vi "test_Parse FPGA Bitfile.vi"(8 "error in (no error)":errorcluster) -> (0 "error out":errorcluster)   [LabVIEW 2018, in "Load And Parse Bitfile Testing.lvclass"]
uses:
  Load And Parse Bitfile Testing.lvclass
  <vilib>/rvi/Bitfile/nirviControlStructure.ctl
  <vilib>/rvi/Bitfile/nirviTypdefDescription.ctl
  <vilib>/rvi/Bitfile/nirviMechanicalAction.ctl
  <vilib>/rvi/Bitfile/nirviSubControlStructure.ctl
  <vilib>/rvi/Bitfile/nirviClusterElementControl.ctl
  <vilib>/rvi/FIFO/Fifo_Types/Fifo_DMA_Config.ctl
  <vilib>/rvi/DataTransferAndStorage/Container/Common/niFpgaDataTypeControl.ctl
  <vilib>/rvi/ClientSDK/Core/ModuleGeneration/CommunicationInterfaceUtility/niFpgaDmaChannelImplementation.ctl
  <vilib>/addons/_JKI Toolkits/VI Tester/TestCase.llb/TestCase.lvclass
  Addon/Addon System Explorer/FPGA Addon System Explorer.lvlib
  C:/Program Files (x86)/National Instruments/LabVIEW 2018/vi.lib/addons/_JKI Toolkits/VI Tester/TestCase.llb/TestCase.lvclass
panel:
  out "TestCase out":refnum<class "Load And Parse Bitfile Testing.lvclass">
  in  "TestCase in":refnum<class "Load And Parse Bitfile Testing.lvclass">
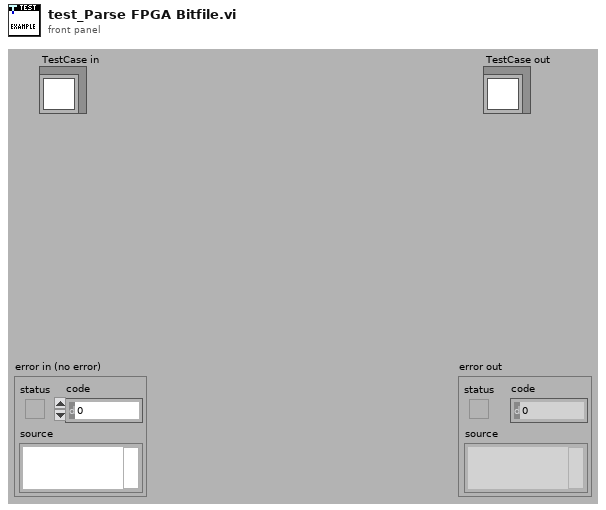
[diagram p1: front panel]
types:
  T1 = typedef "Fifo_DMA_Config.ctl" = cluster{"Name":string, "Depth":u32, "Write? (Deprecated:Use Implementation)":bool, "Physical Channel":u32, "Base Address":u32, "Data Width":u32, "Data Type":T2, "FXP Properties":variant, "Write Window Address":u32, "Implementation":T3, "Control Set":u32}
  T2 = typedef "niFpgaDataTypeControl.ctl" = enum32{"Boolean", "I8", "I16", "I32", "I64", "U8", "U16", "U32", "U64", "FXP", "CustomControl", "SGL"}
  T3 = typedef "niFpgaDmaChannelImplementation.ctl" = enum16{"niFpgaTargetToHost", "niFpgaHostToTarget", "niFpgaPeerToPeerWriter", "niFpgaPeerToPeerReader", "niCoreTargetToHost", "niCoreHostToTarget"}
  T4 = typedef "nirviControlStructure.ctl" = cluster{"Name":string, "Hidden":bool, "Indicator":bool, "Flattened Type":string, "Grouping":cluster{"Grouped":bool, "Member Names":string[], "Member IDs":u32[]}, "Address":u32, "Size":u32, "Class":u32, "Internal":bool, "Typedef":T5, "ID":u32, "Bidirectional":bool, "Synchronous":bool, "Mechanical Action":T6, "Sub Controls":T7[], "Access May Timeout":bool, "Register Node":bool}
  T5 = typedef "nirviTypdefDescription.ctl" = cluster{"Typedef":bool, "Path":path}
  T6 = typedef "nirviMechanicalAction.ctl" = enum8{"Switch When Pressed", "Switch When Released", "Switch Until Released", "Latch When Pressed", "Latch When Released", "Latch Until Released"}
  T7 = typedef "nirviSubControlStructure.ctl" = cluster{"Name":string, "flattened Type":string, "Cluster Information":T8, "Typedef":T5}
  T8 = typedef "nirviClusterElementControl.ctl" = cluster{"Name Hierarchy":string[], "Item Order":u32[]}
  T9 = typedef "niFpgaBitfileStructure_VI.ctl" = cluster{"Name":string, "RegisterMap":T4[], "Icon":T10}
  T10 = typedef "imagedata.ctl" = cluster{"image type":i32, "image depth":i32, "image":u8[], "mask":u8[], "colors":u32[], "Rectangle":cluster{"left":i16, "top":i16, "right":i16, "bottom":i16}}
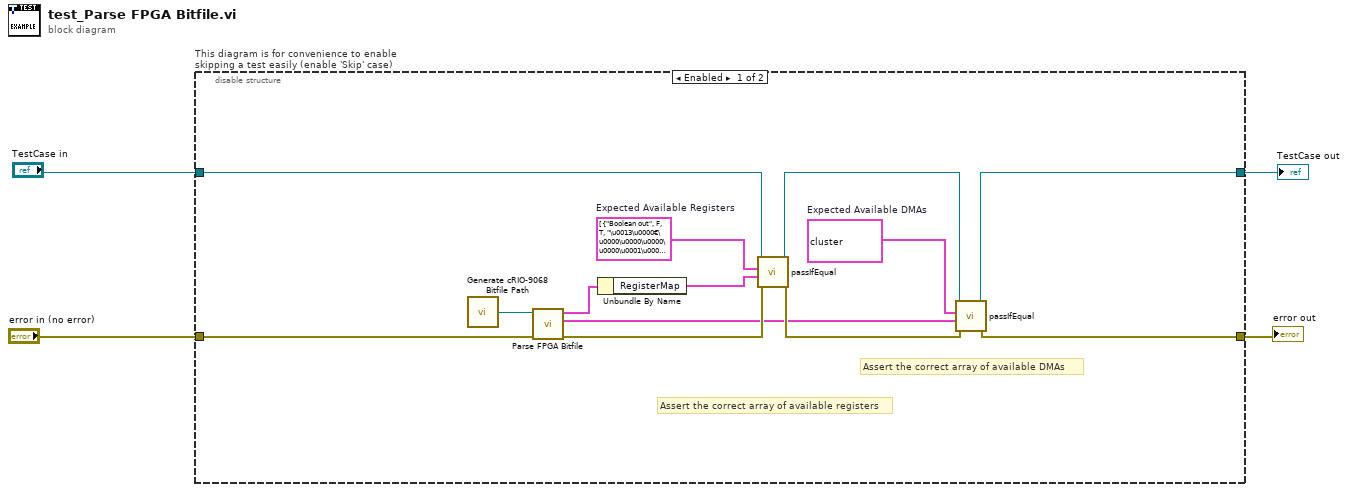
[diagram p0: block diagram]
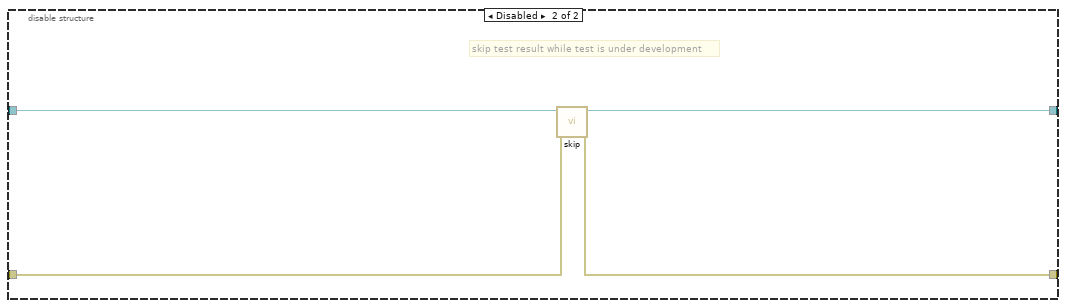
[diagram p2: hidden frame]
diagram:
  n1 = disable-structure "This diagram is for convenience to enable skipping a test easily (enable 'Skip' case)" shown="Enabled" {
    disable-tunnel: "TestCase in" -> [w17 w21]
    disable-tunnel: [w12 w19] -> w1
    disable-tunnel: [w10 w20] -> w3
    disable-tunnel: "error in (no error)" -> [w16 w18]
    frame Enabled {
      w7 = T1[] [{"Name"="Slow", "Depth"=1023, "Write? (Deprecated:Use Implementation)"=TRUE, "Physical Channel"=0, "Base Address"=65472, "Data Width"=32, "Data Type"=enum."SGL", "FXP Properties"=variant(fxp<+/-,32,0> 0.0), "Write Window Address"=0, "Implementation"=enum."niFpgaTargetToHost", "Control Set"=0}, {"Name"="Medium", "Depth"=1023, "Write? (Deprecated:Use Implementation)"=TRUE, "Physical Channel"=1, "Base Address"=65408, "Data Width"=32, "Data Type"=enum."SGL", "FXP Properties"=variant(fxp<+/-,32,0> 0.0), "Write Window Address"=0, "Implementation"=enum."niFpgaTargetToHost", "Control Set"=1}, {"Name"="HostToTarget2", "Depth"=1029, "Write? (Deprecated:Use Implementation)"=FALSE, "Physical Channel"=2, "Base Address"=65344, "Data Width"=32, "Data Type"=enum."SGL", "FXP Properties"=variant(fxp<+/-,32,0> 0.0), "Write Window Address"=0, "Implementation"=enum."niFpgaHostToTarget", "Control Set"=2}, {"Name"="HostToTarget1", "Depth"=1029, "Write? (Deprecated:Use Implementation)"=FALSE, "Physical Channel"=3, "Base Address"=65280, "Data Width"=32, "Data Type"=enum."SGL", "FXP Properties"=variant(fxp<+/-,32,0> 0.0), "Write Window Address"=0, "Implementation"=enum."niFpgaHostToTarget", "Control Set"=3}, {"Name"="Fast", "Depth"=1023, "Write? (Deprecated:Use Implementation)"=TRUE, "Physical Channel"=4, "Base Address"=65216, "Data Width"=32, "Data Type"=enum."SGL", "FXP Properties"=variant(fxp<+/-,32,0> 0.0), "Write Window Address"=0, "Implementation"=enum."niFpgaTargetToHost", "Control Set"=4}]  # Expected Available DMAs
      w6 = T4[] [{"Name"="Boolean out", "Hidden"=FALSE, "Indicator"=TRUE, "Flattened Type"="\u0013\u0000€\u0000\u0000\u0000\u0000\u0001\u0000\u0010@!\u000bBoolean out\u0000\u0001\u0000\u0000\u0000\u0000\u0000\u0000\u0000", "Grouping"={"Grouped"=FALSE, "Member Names"=[], "Member IDs"=[]}, "Address"=98306, "Size"=1, "Class"=8, "Internal"=FALSE, "Typedef"={"Typedef"=FALSE, "Path"=path ""}, "ID"=0, "Bidirectional"=TRUE, "Synchronous"=FALSE, "Mechanical Action"=enum."Switch When Pressed", "Sub Controls"=[], "Access May Timeout"=FALSE, "Register Node"=FALSE}, {"Name"="SGL out", "Hidden"=FALSE, "Indicator"=TRUE, "Flattened Type"="\u0013\u0000€\u0000\u0000\u0000\u0000\u0001\u0000\r@\t\u0000\u0007SGL out\u0000\u0001\u0000\u0000\u0000\u0000\u0000\u0000\u0000\u0000\u0000\u0000", "Grouping"={"Grouped"=FALSE, "Member Names"=[], "Member IDs"=[]}, "Address"=98308, "Size"=32, "Class"=18, "Internal"=FALSE, "Typedef"={"Typedef"=FALSE, "Path"=path ""}, "ID"=1, "Bidirectional"=TRUE, "Synchronous"=FALSE, "Mechanical Action"=enum."Switch When Pressed", "Sub Controls"=[], "Access May Timeout"=FALSE, "Register Node"=FALSE}, {"Name"="U32 out", "Hidden"=FALSE, "Indicator"=TRUE, "Flattened Type"="\u0013\u0000€\u0000\u0000\u0000\u0000\u0001\u0000\r@\u0007\u0000\u0007U32 out\u0000\u0001\u0000\u0000\u0000\u0000\u0000\u0000\u0000\u0000\u0000\u0000", "Grouping"={"Grouped"=FALSE, "Member Names"=[], "Member IDs"=[]}, "Address"=98312, "Size"=32, "Class"=18, "Internal"=FALSE, "Typedef"={"Typedef"=FALSE, "Path"=path ""}, "ID"=2, "Bidirectional"=TRUE, "Synchronous"=FALSE, "Mechanical Action"=enum."Switch When Pressed", "Sub Controls"=[], "Access May Timeout"=FALSE, "Register Node"=FALSE}, {"Name"="U64 out", "Hidden"=FALSE, "Indicator"=TRUE, "Flattened Type"="\u0013\u0000€\u0000\u0000\u0000\u0000\u0001\u0000\r@\b\u0000\u0007U64 out\u0000\u0001\u0000\u0000\u0000\u0000\u0000\u0000\u0000\u0000\u0000\u0000\u0000\u0000\u0000\u0000", "Grouping"={"Grouped"=FALSE, "Member Names"=[], "Member IDs"=[]}, "Address"=98316, "Size"=64, "Class"=18, "Internal"=FALSE, "Typedef"={"Typedef"=FALSE, "Path"=path ""}, "ID"=3, "Bidirectional"=TRUE, "Synchronous"=FALSE, "Mechanical Action"=enum."Switch When Pressed", "Sub Controls"=[], "Access May Timeout"=FALSE, "Register Node"=FALSE}, {"Name"="U8 out", "Hidden"=FALSE, "Indicator"=TRUE, "Flattened Type"="\u0013\u0000€\u0000\u0000\u0000\u0000\u0001\u0000\r@\u0005\u0000\u0006U8 out\u0000\u0000\u0001\u0000\u0000\u0000\u0000\u0000\u0000\u0000", "Grouping"={"Grouped"=FALSE, "Member Names"=[], "Member IDs"=[]}, "Address"=98322, "Size"=8, "Class"=18, "Internal"=FALSE, "Typedef"={"Typedef"=FALSE, "Path"=path ""}, "ID"=4, "Bidirectional"=TRUE, "Synchronous"=FALSE, "Mechanical Action"=enum."Switch When Pressed", "Sub Controls"=[], "Access May Timeout"=FALSE, "Register Node"=FALSE}, {"Name"="U16 out", "Hidden"=FALSE, "Indicator"=TRUE, "Flattened Type"="\u0013\u0000€\u0000\u0000\u0000\u0000\u0001\u0000\r@\u0006\u0000\u0007U16 out\u0000\u0001\u0000\u0000\u0000\u0000\u0000\u0000\u0000\u0000", "Grouping"={"Grouped"=FALSE, "Member Names"=[], "Member IDs"=[]}, "Address"=98326, "Size"=16, "Class"=18, "Internal"=FALSE, "Typedef"={"Typedef"=FALSE, "Path"=path ""}, "ID"=5, "Bidirectional"=TRUE, "Synchronous"=FALSE, "Mechanical Action"=enum."Switch When Pressed", "Sub Controls"=[], "Access May Timeout"=FALSE, "Register Node"=FALSE}, {"Name"="I32 out", "Hidden"=FALSE, "Indicator"=TRUE, "Flattened Type"="\u0013\u0000€\u0000\u0000\u0000\u0000\u0001\u0000\r@\u0003\u0000\u0007I32 out\u0000\u0001\u0000\u0000\u0000\u0000\u0000\u0000\u0000\u0000\u0000\u0000", "Grouping"={"Grouped"=FALSE, "Member Names"=[], "Member IDs"=[]}, "Address"=98328, "Size"=32, "Class"=18, "Internal"=FALSE, "Typedef"={"Typedef"=FALSE, "Path"=path ""}, "ID"=6, "Bidirectional"=TRUE, "Synchronous"=FALSE, "Mechanical Action"=enum."Switch When Pressed", "Sub Controls"=[], "Access May Timeout"=FALSE, "Register Node"=FALSE}, {"Name"="I64 out", "Hidden"=FALSE, "Indicator"=TRUE, "Flattened Type"="\u0013\u0000€\u0000\u0000\u0000\u0000\u0001\u0000\r@\u0004\u0000\u0007I64 out\u0000\u0001\u0000\u0000\u0000\u0000\u0000\u0000\u0000\u0000\u0000\u0000\u0000\u0000\u0000\u0000", "Grouping"={"Grouped"=FALSE, "Member Names"=[], "Member IDs"=[]}, "Address"=98332, "Size"=64, "Class"=18, "Internal"=FALSE, "Typedef"={"Typedef"=FALSE, "Path"=path ""}, "ID"=7, "Bidirectional"=TRUE, "Synchronous"=FALSE, "Mechanical Action"=enum."Switch When Pressed", "Sub Controls"=[], "Access May Timeout"=FALSE, "Register Node"=FALSE}, {"Name"="I8 out", "Hidden"=FALSE, "Indicator"=TRUE, "Flattened Type"="\u0013\u0000€\u0000\u0000\u0000\u0000\u0001\u0000\r@\u0001\u0000\u0006I8 out\u0000\u0000\u0001\u0000\u0000\u0000\u0000\u0000\u0000\u0000", "Grouping"={"Grouped"=FALSE, "Member Names"=[], "Member IDs"=[]}, "Address"=98338, "Size"=8, "Class"=18, "Internal"=FALSE, "Typedef"={"Typedef"=FALSE, "Path"=path ""}, "ID"=8, "Bidirectional"=TRUE, "Synchronous"=FALSE, "Mechanical Action"=enum."Switch When Pressed", "Sub Controls"=[], "Access May Timeout"=FALSE, "Register Node"=FALSE}, {"Name"="I16 out", "Hidden"=FALSE, "Indicator"=TRUE, "Flattened Type"="\u0013\u0000€\u0000\u0000\u0000\u0000\u0001\u0000\r@\u0002\u0000\u0007I16 out\u0000\u0001\u0000\u0000\u0000\u0000\u0000\u0000\u0000\u0000", "Grouping"={"Grouped"=FALSE, "Member Names"=[], "Member IDs"=[]}, "Address"=98342, "Size"=16, "Class"=18, "Internal"=FALSE, "Typedef"={"Typedef"=FALSE, "Path"=path ""}, "ID"=9, "Bidirectional"=TRUE, "Synchronous"=FALSE, "Mechanical Action"=enum."Switch When Pressed", "Sub Controls"=[], "Access May Timeout"=FALSE, "Register Node"=FALSE}, {"Name"="Boolean", "Hidden"=FALSE, "Indicator"=FALSE, "Flattened Type"="\u0013\u0000€\u0000\u0000\u0000\u0000\u0001\u0000\f@!\u0007Boolean\u0000\u0001\u0000\u0000\u0000\u0000\u0000\u0000\u0000", "Grouping"={"Grouped"=FALSE, "Member Names"=[], "Member IDs"=[]}, "Address"=98346, "Size"=1, "Class"=8, "Internal"=FALSE, "Typedef"={"Typedef"=FALSE, "Path"=path ""}, "ID"=10, "Bidirectional"=TRUE, "Synchronous"=FALSE, "Mechanical Action"=enum."Switch When Pressed", "Sub Controls"=[], "Access May Timeout"=FALSE, "Register Node"=FALSE}, {"Name"="SGL", "Hidden"=FALSE, "Indicator"=FALSE, "Flattened Type"="\u0013\u0000€\u0000\u0000\u0000\u0000\u0001\u0000\t@\t\u0000\u0003SGL\u0000\u0001\u0000\u0000\u0000\u0000\u0000\u0000\u0000\u0000\u0000\u0000", "Grouping"={"Grouped"=FALSE, "Member Names"=[], "Member IDs"=[]}, "Address"=98348, "Size"=32, "Class"=18, "Internal"=FALSE, "Typedef"={"Typedef"=FALSE, "Path"=path ""}, "ID"=11, "Bidirectional"=TRUE, "Synchronous"=FALSE, "Mechanical Action"=enum."Switch When Pressed", "Sub Controls"=[], "Access May Timeout"=FALSE, "Register Node"=FALSE}, {"Name"="U32", "Hidden"=FALSE, "Indicator"=FALSE, "Flattened Type"="\u0013\u0000€\u0000\u0000\u0000\u0000\u0001\u0000\t@\u0007\u0000\u0003U32\u0000\u0001\u0000\u0000\u0000\u0000\u0000\u0000\u0000\u0000\u0000\u0000", "Grouping"={"Grouped"=FALSE, "Member Names"=[], "Member IDs"=[]}, "Address"=98352, "Size"=32, "Class"=18, "Internal"=FALSE, "Typedef"={"Typedef"=FALSE, "Path"=path ""}, "ID"=12, "Bidirectional"=TRUE, "Synchronous"=FALSE, "Mechanical Action"=enum."Switch When Pressed", "Sub Controls"=[], "Access May Timeout"=FALSE, "Register Node"=FALSE}, {"Name"="U64", "Hidden"=FALSE, "Indicator"=FALSE, "Flattened Type"="\u0013\u0000€\u0000\u0000\u0000\u0000\u0001\u0000\t@\b\u0000\u0003U64\u0000\u0001\u0000\u0000\u0000\u0000\u0000\u0000\u0000\u0000\u0000\u0000\u0000\u0000\u0000\u0000", "Grouping"={"Grouped"=FALSE, "Member Names"=[], "Member IDs"=[]}, "Address"=98356, "Size"=64, "Class"=18, "Internal"=FALSE, "Typedef"={"Typedef"=FALSE, "Path"=path ""}, "ID"=13, "Bidirectional"=TRUE, "Synchronous"=FALSE, "Mechanical Action"=enum."Switch When Pressed", "Sub Controls"=[], "Access May Timeout"=FALSE, "Register Node"=FALSE}, {"Name"="U8", "Hidden"=FALSE, "Indicator"=FALSE, "Flattened Type"="\u0013\u0000€\u0000\u0000\u0000\u0000\u0001\u0000\t@\u0005\u0000\u0002U8\u0000\u0000\u0001\u0000\u0000\u0000\u0000\u0000\u0000\u0000", "Grouping"={"Grouped"=FALSE, "Member Names"=[], "Member IDs"=[]}, "Address"=98362, "Size"=8, "Class"=18, "Internal"=FALSE, "Typedef"={"Typedef"=FALSE, "Path"=path ""}, "ID"=14, "Bidirectional"=TRUE, "Synchronous"=FALSE, "Mechanical Action"=enum."Switch When Pressed", "Sub Controls"=[], "Access May Timeout"=FALSE, "Register Node"=FALSE}, {"Name"="U16", "Hidden"=FALSE, "Indicator"=FALSE, "Flattened Type"="\u0013\u0000€\u0000\u0000\u0000\u0000\u0001\u0000\t@\u0006\u0000\u0003U16\u0000\u0001\u0000\u0000\u0000\u0000\u0000\u0000\u0000\u0000", "Grouping"={"Grouped"=FALSE, "Member Names"=[], "Member IDs"=[]}, "Address"=98366, "Size"=16, "Class"=18, "Internal"=FALSE, "Typedef"={"Typedef"=FALSE, "Path"=path ""}, "ID"=15, "Bidirectional"=TRUE, "Synchronous"=FALSE, "Mechanical Action"=enum."Switch When Pressed", "Sub Controls"=[], "Access May Timeout"=FALSE, "Register Node"=FALSE}, {"Name"="I32", "Hidden"=FALSE, "Indicator"=FALSE, "Flattened Type"="\u0013\u0000€\u0000\u0000\u0000\u0000\u0001\u0000\t@\u0003\u0000\u0003I32\u0000\u0001\u0000\u0000\u0000\u0000\u0000\u0000\u0000\u0000\u0000\u0000", "Grouping"={"Grouped"=FALSE, "Member Names"=[], "Member IDs"=[]}, "Address"=98368, "Size"=32, "Class"=18, "Internal"=FALSE, "Typedef"={"Typedef"=FALSE, "Path"=path ""}, "ID"=16, "Bidirectional"=TRUE, "Synchronous"=FALSE, "Mechanical Action"=enum."Switch When Pressed", "Sub Controls"=[], "Access May Timeout"=FALSE, "Register Node"=FALSE}, {"Name"="I64", "Hidden"=FALSE, "Indicator"=FALSE, "Flattened Type"="\u0013\u0000€\u0000\u0000\u0000\u0000\u0001\u0000\t@\u0004\u0000\u0003I64\u0000\u0001\u0000\u0000\u0000\u0000\u0000\u0000\u0000\u0000\u0000\u0000\u0000\u0000\u0000\u0000", "Grouping"={"Grouped"=FALSE, "Member Names"=[], "Member IDs"=[]}, "Address"=98372, "Size"=64, "Class"=18, "Internal"=FALSE, "Typedef"={"Typedef"=FALSE, "Path"=path ""}, "ID"=17, "Bidirectional"=TRUE, "Synchronous"=FALSE, "Mechanical Action"=enum."Switch When Pressed", "Sub Controls"=[], "Access May Timeout"=FALSE, "Register Node"=FALSE}, {"Name"="I8", "Hidden"=FALSE, "Indicator"=FALSE, "Flattened Type"="\u0013\u0000€\u0000\u0000\u0000\u0000\u0001\u0000\t@\u0001\u0000\u0002I8\u0000\u0000\u0001\u0000\u0000\u0000\u0000\u0000\u0000\u0000", "Grouping"={"Grouped"=FALSE, "Member Names"=[], "Member IDs"=[]}, "Address"=98378, "Size"=8, "Class"=18, "Internal"=FALSE, "Typedef"={"Typedef"=FALSE, "Path"=path ""}, "ID"=18, "Bidirectional"=TRUE, "Synchronous"=FALSE, "Mechanical Action"=enum."Switch When Pressed", "Sub Controls"=[], "Access May Timeout"=FALSE, "Register Node"=FALSE}, {"Name"="I16", "Hidden"=FALSE, "Indicator"=FALSE, "Flattened Type"="\u0013\u0000€\u0000\u0000\u0000\u0000\u0001\u0000\t@\u0002\u0000\u0003I16\u0000\u0001\u0000\u0000\u0000\u0000\u0000\u0000\u0000\u0000", "Grouping"={"Grouped"=FALSE, "Member Names"=[], "Member IDs"=[]}, "Address"=98382, "Size"=16, "Class"=18, "Internal"=FALSE, "Typedef"={"Typedef"=FALSE, "Path"=path ""}, "ID"=19, "Bidirectional"=TRUE, "Synchronous"=FALSE, "Mechanical Action"=enum."Switch When Pressed", "Sub Controls"=[], "Access May Timeout"=FALSE, "Register Node"=FALSE}, {"Name"="Slow timeout", "Hidden"=FALSE, "Indicator"=TRUE, "Flattened Type"="\u0013\u0000€\u0000\u0000\u0000\u0000\u0001\u0000\u0012@!\fSlow timeout\u0000\u0000\u0001\u0000\u0000\u0000\u0000\u0000\u0000\u0000", "Grouping"={"Grouped"=FALSE, "Member Names"=[], "Member IDs"=[]}, "Address"=98386, "Size"=1, "Class"=8, "Internal"=FALSE, "Typedef"={"Typedef"=FALSE, "Path"=path ""}, "ID"=20, "Bidirectional"=TRUE, "Synchronous"=FALSE, "Mechanical Action"=enum."Switch When Pressed", "Sub Controls"=[], "Access May Timeout"=FALSE, "Register Node"=FALSE}, {"Name"="Med timeout", "Hidden"=FALSE, "Indicator"=TRUE, "Flattened Type"="\u0013\u0000€\u0000\u0000\u0000\u0000\u0001\u0000\u0010@!\u000bMed timeout\u0000\u0001\u0000\u0000\u0000\u0000\u0000\u0000\u0000", "Grouping"={"Grouped"=FALSE, "Member Names"=[], "Member IDs"=[]}, "Address"=98390, "Size"=1, "Class"=8, "Internal"=FALSE, "Typedef"={"Typedef"=FALSE, "Path"=path ""}, "ID"=21, "Bidirectional"=TRUE, "Synchronous"=FALSE, "Mechanical Action"=enum."Switch When Pressed", "Sub Controls"=[], "Access May Timeout"=FALSE, "Register Node"=FALSE}, {"Name"="Fast timeout", "Hidden"=FALSE, "Indicator"=TRUE, "Flattened Type"="\u0013\u0000€\u0000\u0000\u0000\u0000\u0001\u0000\u0012@!\fFast timeout\u0000\u0000\u0001\u0000\u0000\u0000\u0000\u0000\u0000\u0000", "Grouping"={"Grouped"=FALSE, "Member Names"=[], "Member IDs"=[]}, "Address"=98394, "Size"=1, "Class"=8, "Internal"=FALSE, "Typedef"={"Typedef"=FALSE, "Path"=path ""}, "ID"=22, "Bidirectional"=TRUE, "Synchronous"=FALSE, "Mechanical Action"=enum."Switch When Pressed", "Sub Controls"=[], "Access May Timeout"=FALSE, "Register Node"=FALSE}, {"Name"="FXP24.5", "Hidden"=FALSE, "Indicator"=FALSE, "Flattened Type"="\u0013\u0000€\u0000\u0000\u0000\u0000\u0001\u0000D@_\u0003Q\u0000\u0018\u0000\u0000\u0000\u0005\u0000\u0001\u0000\u0001\u0000\u0000\u0000\u0005ÿÿÿÿÿÿÿÿ\u0000\u0000\u0000\u0017\u0000\u0000\u0000\u0004\u0000\u0000\u0000\u0000\u0000ÿÿ\u0000\u0000\u0000\u0001ÿÿÿî\u0000\u0000\u0000\u0000\u0000\u0000\u0000\u0001\u0007FXP24.5\u0000\u0001\u0000\u0000\u0000\u0000\u0000\u0000\u0000\u0000\u0000\u0000\u0000\u0000\u0000\u0000", "Grouping"={"Grouped"=FALSE, "Member Names"=[], "Member IDs"=[]}, "Address"=98396, "Size"=24, "Class"=18, "Internal"=FALSE, "Typedef"={"Typedef"=FALSE, "Path"=path ""}, "ID"=23, "Bidirectional"=TRUE, "Synchronous"=FALSE, "Mechanical Action"=enum."Switch When Pressed", "Sub Controls"=[], "Access May Timeout"=FALSE, "Register Node"=FALSE}, {"Name"="FXP16.5", "Hidden"=FALSE, "Indicator"=FALSE, "Flattened Type"="\u0013\u0000€\u0000\u0000\u0000\u0000\u0001\u0000D@_\u0003Q\u0000\u0010\u0000\u0000\u0000\u0005\u0000\u0001\u0000\u0001\u0000\u0000\u0000\u0005ÿÿÿÿÿÿÿÿ\u0000\u0000\u0000\u000f\u0000\u0000\u0000\u0004\u0000\u0000\u0000\u0000\u0000\u0000ÿ\u0000\u0000\u0000\u0001ÿÿÿö\u0000\u0000\u0000\u0000\u0000\u0000\u0000\u0001\u0007FXP16.5\u0000\u0001\u0000\u0000\u0000\u0000\u0000\u0000\u0000\u0000\u0000\u0000\u0000\u0000\u0000\u0000", "Grouping"={"Grouped"=FALSE, "Member Names"=[], "Member IDs"=[]}, "Address"=98402, "Size"=16, "Class"=18, "Internal"=FALSE, "Typedef"={"Typedef"=FALSE, "Path"=path ""}, "ID"=24, "Bidirectional"=TRUE, "Synchronous"=FALSE, "Mechanical Action"=enum."Switch When Pressed", "Sub Controls"=[], "Access May Timeout"=FALSE, "Register Node"=FALSE}, {"Name"="FXP32.8", "Hidden"=FALSE, "Indicator"=FALSE, "Flattened Type"="\u0013\u0000€\u0000\u0000\u0000\u0000\u0001\u0000D@_\u0003Q\u0000 \u0000\u0000\u0000\b\u0000\u0001\u0000\u0001\u0000\u0000\u0000\bÿÿÿÿÿÿÿÿ\u0000\u0000\u0000\u001f\u0000\u0000\u0000\u0007\u0000\u0000\u0000\u0000ÿÿÿ\u0000\u0000\u0000\u0001ÿÿÿé\u0000\u0000\u0000\u0000\u0000\u0000\u0000\u0001\u0007FXP32.8\u0000\u0001\u0000\u0000\u0000\u0000\u0000\u0000\u0000\u0000\u0000\u0000\u0000\u0000\u0000\u0000", "Grouping"={"Grouped"=FALSE, "Member Names"=[], "Member IDs"=[]}, "Address"=98404, "Size"=32, "Class"=18, "Internal"=FALSE, "Typedef"={"Typedef"=FALSE, "Path"=path ""}, "ID"=25, "Bidirectional"=TRUE, "Synchronous"=FALSE, "Mechanical Action"=enum."Switch When Pressed", "Sub Controls"=[], "Access May Timeout"=FALSE, "Register Node"=FALSE}, {"Name"="FXP64.32", "Hidden"=FALSE, "Indicator"=FALSE, "Flattened Type"="\u0013\u0000€\u0000\u0000\u0000\u0000\u0001\u0000F@_\u0003Q\u0000@\u0000\u0000\u0000 \u0000\u0001\u0000\u0001\u0000\u0000\u0000 ÿÿÿÿÿÿÿÿ\u0000\u0000\u0000?\u0000\u0000\u0000\u001fÿÿÿÿÿÿÿ\u0000\u0000\u0000\u0001ÿÿÿá\u0000\u0000\u0000\u0000\u0000\u0000\u0000\u0001\bFXP64.32\u0000\u0000\u0001\u0000\u0000\u0000\u0000\u0000\u0000\u0000\u0000\u0000\u0000\u0000\u0000\u0000\u0000", "Grouping"={"Grouped"=FALSE, "Member Names"=[], "Member IDs"=[]}, "Address"=98408, "Size"=64, "Class"=18, "Internal"=FALSE, "Typedef"={"Typedef"=FALSE, "Path"=path ""}, "ID"=26, "Bidirectional"=TRUE, "Synchronous"=FALSE, "Mechanical Action"=enum."Switch When Pressed", "Sub Controls"=[], "Access May Timeout"=FALSE, "Register Node"=FALSE}, {"Name"="FXP24.5 out", "Hidden"=FALSE, "Indicator"=TRUE, "Flattened Type"="\u0013\u0000€\u0000\u0000\u0000\u0000\u0001\u0000H@_\u0003Q\u0000\u0018\u0000\u0000\u0000\u0005\u0000\u0001\u0000\u0001\u0000\u0000\u0000\u0005ÿÿÿÿÿÿÿÿ\u0000\u0000\u0000\u0017\u0000\u0000\u0000\u0004\u0000\u0000\u0000\u0000\u0000ÿÿ\u0000\u0000\u0000\u0001ÿÿÿî\u0000\u0000\u0000\u0000\u0000\u0000\u0000\u0001\u000bFXP24.5 out\u0000\u0001\u0000\u0000\u0000\u0000\u0000\u0000\u0000\u0000\u0000\u0000\u0000\u0000\u0000\u0000", "Grouping"={"Grouped"=FALSE, "Member Names"=[], "Member IDs"=[]}, "Address"=98412, "Size"=24, "Class"=18, "Internal"=FALSE, "Typedef"={"Typedef"=FALSE, "Path"=path ""}, "ID"=27, "Bidirectional"=TRUE, "Synchronous"=FALSE, "Mechanical Action"=enum."Switch When Pressed", "Sub Controls"=[], "Access May Timeout"=FALSE, "Register Node"=FALSE}, {"Name"="FXP16.5 out", "Hidden"=FALSE, "Indicator"=TRUE, "Flattened Type"="\u0013\u0000€\u0000\u0000\u0000\u0000\u0001\u0000H@_\u0003Q\u0000\u0010\u0000\u0000\u0000\u0005\u0000\u0001\u0000\u0001\u0000\u0000\u0000\u0005ÿÿÿÿÿÿÿÿ\u0000\u0000\u0000\u000f\u0000\u0000\u0000\u0004\u0000\u0000\u0000\u0000\u0000\u0000ÿ\u0000\u0000\u0000\u0001ÿÿÿö\u0000\u0000\u0000\u0000\u0000\u0000\u0000\u0001\u000bFXP16.5 out\u0000\u0001\u0000\u0000\u0000\u0000\u0000\u0000\u0000\u0000\u0000\u0000\u0000\u0000\u0000\u0000", "Grouping"={"Grouped"=FALSE, "Member Names"=[], "Member IDs"=[]}, "Address"=98418, "Size"=16, "Class"=18, "Internal"=FALSE, "Typedef"={"Typedef"=FALSE, "Path"=path ""}, "ID"=28, "Bidirectional"=TRUE, "Synchronous"=FALSE, "Mechanical Action"=enum."Switch When Pressed", "Sub Controls"=[], "Access May Timeout"=FALSE, "Register Node"=FALSE}, {"Name"="FXP32.8 out", "Hidden"=FALSE, "Indicator"=TRUE, "Flattened Type"="\u0013\u0000€\u0000\u0000\u0000\u0000\u0001\u0000H@_\u0003Q\u0000 \u0000\u0000\u0000\b\u0000\u0001\u0000\u0001\u0000\u0000\u0000\bÿÿÿÿÿÿÿÿ\u0000\u0000\u0000\u001f\u0000\u0000\u0000\u0007\u0000\u0000\u0000\u0000ÿÿÿ\u0000\u0000\u0000\u0001ÿÿÿé\u0000\u0000\u0000\u0000\u0000\u0000\u0000\u0001\u000bFXP32.8 out\u0000\u0001\u0000\u0000\u0000\u0000\u0000\u0000\u0000\u0000\u0000\u0000\u0000\u0000\u0000\u0000", "Grouping"={"Grouped"=FALSE, "Member Names"=[], "Member IDs"=[]}, "Address"=98420, "Size"=32, "Class"=18, "Internal"=FALSE, "Typedef"={"Typedef"=FALSE, "Path"=path ""}, "ID"=29, "Bidirectional"=TRUE, "Synchronous"=FALSE, "Mechanical Action"=enum."Switch When Pressed", "Sub Controls"=[], "Access May Timeout"=FALSE, "Register Node"=FALSE}, {"Name"="FXP64.32 out", "Hidden"=FALSE, "Indicator"=TRUE, "Flattened Type"="\u0013\u0000€\u0000\u0000\u0000\u0000\u0001\u0000J@_\u0003Q\u0000@\u0000\u0000\u0000 \u0000\u0001\u0000\u0001\u0000\u0000\u0000 ÿÿÿÿÿÿÿÿ\u0000\u0000\u0000?\u0000\u0000\u0000\u001fÿÿÿÿÿÿÿ\u0000\u0000\u0000\u0001ÿÿÿá\u0000\u0000\u0000\u0000\u0000\u0000\u0000\u0001\fFXP64.32 out\u0000\u0000\u0001\u0000\u0000\u0000\u0000\u0000\u0000\u0000\u0000\u0000\u0000\u0000\u0000\u0000\u0000", "Grouping"={"Grouped"=FALSE, "Member Names"=[], "Member IDs"=[]}, "Address"=98424, "Size"=64, "Class"=18, "Internal"=FALSE, "Typedef"={"Typedef"=FALSE, "Path"=path ""}, "ID"=30, "Bidirectional"=TRUE, "Synchronous"=FALSE, "Mechanical Action"=enum."Switch When Pressed", "Sub Controls"=[], "Access May Timeout"=FALSE, "Register Node"=FALSE}, {"Name"="FXP16.7 out", "Hidden"=FALSE, "Indicator"=TRUE, "Flattened Type"="\u0013\u0000€\u0000\u0000\u0000\u0000\u0001\u0000H@_\u0003Q\u0000\u0010\u0000\u0000\u0000\u0007\u0000\u0001\u0000\u0001\u0000\u0000\u0000\u0007ÿÿÿÿÿÿÿÿ\u0000\u0000\u0000\u000f\u0000\u0000\u0000\u0006\u0000\u0000\u0000\u0000\u0000\u0000ÿ\u0000\u0000\u0000\u0001ÿÿÿø\u0000\u0000\u0000\u0000\u0000\u0000\u0000\u0001\u000bFXP16.7 out\u0000\u0001\u0000\u0000\u0000\u0000\u0000\u0000\u0000\u0000\u0000\u0000\u0000\u0000\u0000\u0000", "Grouping"={"Grouped"=FALSE, "Member Names"=[], "Member IDs"=[]}, "Address"=98430, "Size"=16, "Class"=18, "Internal"=FALSE, "Typedef"={"Typedef"=FALSE, "Path"=path ""}, "ID"=31, "Bidirectional"=TRUE, "Synchronous"=FALSE, "Mechanical Action"=enum."Switch When Pressed", "Sub Controls"=[], "Access May Timeout"=FALSE, "Register Node"=FALSE}, {"Name"="FXP16.7", "Hidden"=FALSE, "Indicator"=FALSE, "Flattened Type"="\u0013\u0000€\u0000\u0000\u0000\u0000\u0001\u0000D@_\u0003Q\u0000\u0010\u0000\u0000\u0000\u0007\u0000\u0001\u0000\u0001\u0000\u0000\u0000\u0007ÿÿÿÿÿÿÿÿ\u0000\u0000\u0000\u000f\u0000\u0000\u0000\u0006\u0000\u0000\u0000\u0000\u0000\u0000ÿ\u0000\u0000\u0000\u0001ÿÿÿø\u0000\u0000\u0000\u0000\u0000\u0000\u0000\u0001\u0007FXP16.7\u0000\u0001\u0000\u0000\u0000\u0000\u0000\u0000\u0000\u0000\u0000\u0000\u0000\u0000\u0000\u0000", "Grouping"={"Grouped"=FALSE, "Member Names"=[], "Member IDs"=[]}, "Address"=98434, "Size"=16, "Class"=18, "Internal"=FALSE, "Typedef"={"Typedef"=FALSE, "Path"=path ""}, "ID"=32, "Bidirectional"=TRUE, "Synchronous"=FALSE, "Mechanical Action"=enum."Switch When Pressed", "Sub Controls"=[], "Access May Timeout"=FALSE, "Register Node"=FALSE}, {"Name"="FXP20.5 out", "Hidden"=FALSE, "Indicator"=TRUE, "Flattened Type"="\u0013\u0000€\u0000\u0000\u0000\u0000\u0001\u0000H@_\u0003Q\u0000\u0014\u0000\u0000\u0000\u0005\u0000\u0001\u0000\u0001\u0000\u0000\u0000\u0005ÿÿÿÿÿÿÿÿ\u0000\u0000\u0000\u0013\u0000\u0000\u0000\u0004\u0000\u0000\u0000\u0000\u0000\u0007ÿÿ\u0000\u0000\u0000\u0001ÿÿÿò\u0000\u0000\u0000\u0000\u0000\u0000\u0000\u0001\u000bFXP20.5 out\u0000\u0001\u0000\u0000\u0000\u0000\u0000\u0000\u0000\u0000\u0000\u0000\u0000\u0000\u0000\u0000", "Grouping"={"Grouped"=FALSE, "Member Names"=[], "Member IDs"=[]}, "Address"=98436, "Size"=20, "Class"=18, "Internal"=FALSE, "Typedef"={"Typedef"=FALSE, "Path"=path ""}, "ID"=33, "Bidirectional"=TRUE, "Synchronous"=FALSE, "Mechanical Action"=enum."Switch When Pressed", "Sub Controls"=[], "Access May Timeout"=FALSE, "Register Node"=FALSE}, {"Name"="FXP20.5", "Hidden"=FALSE, "Indicator"=FALSE, "Flattened Type"="\u0013\u0000€\u0000\u0000\u0000\u0000\u0001\u0000D@_\u0003Q\u0000\u0014\u0000\u0000\u0000\u0005\u0000\u0001\u0000\u0001\u0000\u0000\u0000\u0005ÿÿÿÿÿÿÿÿ\u0000\u0000\u0000\u0013\u0000\u0000\u0000\u0004\u0000\u0000\u0000\u0000\u0000\u0007ÿÿ\u0000\u0000\u0000\u0001ÿÿÿò\u0000\u0000\u0000\u0000\u0000\u0000\u0000\u0001\u0007FXP20.5\u0000\u0001\u0000\u0000\u0000\u0000\u0000\u0000\u0000\u0000\u0000\u0000\u0000\u0000\u0000\u0000", "Grouping"={"Grouped"=FALSE, "Member Names"=[], "Member IDs"=[]}, "Address"=98440, "Size"=20, "Class"=18, "Internal"=FALSE, "Typedef"={"Typedef"=FALSE, "Path"=path ""}, "ID"=34, "Bidirectional"=TRUE, "Synchronous"=FALSE, "Mechanical Action"=enum."Switch When Pressed", "Sub Controls"=[], "Access May Timeout"=FALSE, "Register Node"=FALSE}, {"Name"="FXP27.5 out", "Hidden"=FALSE, "Indicator"=TRUE, "Flattened Type"="\u0013\u0000€\u0000\u0000\u0000\u0000\u0001\u0000H@_\u0003Q\u0000\u001b\u0000\u0000\u0000\u0005\u0000\u0001\u0000\u0001\u0000\u0000\u0000\u0005ÿÿÿÿÿÿÿÿ\u0000\u0000\u0000\u001a\u0000\u0000\u0000\u0004\u0000\u0000\u0000\u0000\u0003ÿÿÿ\u0000\u0000\u0000\u0001ÿÿÿë\u0000\u0000\u0000\u0000\u0000\u0000\u0000\u0001\u000bFXP27.5 out\u0000\u0001\u0000\u0000\u0000\u0000\u0000\u0000\u0000\u0000\u0000\u0000\u0000\u0000\u0000\u0000", "Grouping"={"Grouped"=FALSE, "Member Names"=[], "Member IDs"=[]}, "Address"=98444, "Size"=27, "Class"=18, "Internal"=FALSE, "Typedef"={"Typedef"=FALSE, "Path"=path ""}, "ID"=35, "Bidirectional"=TRUE, "Synchronous"=FALSE, "Mechanical Action"=enum."Switch When Pressed", "Sub Controls"=[], "Access May Timeout"=FALSE, "Register Node"=FALSE}, {"Name"="FXP27.5", "Hidden"=FALSE, "Indicator"=FALSE, "Flattened Type"="\u0013\u0000€\u0000\u0000\u0000\u0000\u0001\u0000D@_\u0003Q\u0000\u001b\u0000\u0000\u0000\u0005\u0000\u0001\u0000\u0001\u0000\u0000\u0000\u0005ÿÿÿÿÿÿÿÿ\u0000\u0000\u0000\u001a\u0000\u0000\u0000\u0004\u0000\u0000\u0000\u0000\u0003ÿÿÿ\u0000\u0000\u0000\u0001ÿÿÿë\u0000\u0000\u0000\u0000\u0000\u0000\u0000\u0001\u0007FXP27.5\u0000\u0001\u0000\u0000\u0000\u0000\u0000\u0000\u0000\u0000\u0000\u0000\u0000\u0000\u0000\u0000", "Grouping"={"Grouped"=FALSE, "Member Names"=[], "Member IDs"=[]}, "Address"=98448, "Size"=27, "Class"=18, "Internal"=FALSE, "Typedef"={"Typedef"=FALSE, "Path"=path ""}, "ID"=36, "Bidirectional"=TRUE, "Synchronous"=FALSE, "Mechanical Action"=enum."Switch When Pressed", "Sub Controls"=[], "Access May Timeout"=FALSE, "Register Node"=FALSE}, {"Name"="FXP32.16 out", "Hidden"=FALSE, "Indicator"=TRUE, "Flattened Type"="\u0013\u0000€\u0000\u0000\u0000\u0000\u0001\u0000J@_\u0003Q\u0000 \u0000\u0000\u0000\u0010\u0000\u0001\u0000\u0001\u0000\u0000\u0000\u0010ÿÿÿÿÿÿÿÿ\u0000\u0000\u0000\u001f\u0000\u0000\u0000\u000f\u0000\u0000\u0000\u0000ÿÿÿ\u0000\u0000\u0000\u0001ÿÿÿñ\u0000\u0000\u0000\u0000\u0000\u0000\u0000\u0001\fFXP32.16 out\u0000\u0000\u0001\u0000\u0000\u0000\u0000\u0000\u0000\u0000\u0000\u0000\u0000\u0000\u0000\u0000\u0000", "Grouping"={"Grouped"=FALSE, "Member Names"=[], "Member IDs"=[]}, "Address"=98452, "Size"=32, "Class"=18, "Internal"=FALSE, "Typedef"={"Typedef"=FALSE, "Path"=path ""}, "ID"=37, "Bidirectional"=TRUE, "Synchronous"=FALSE, "Mechanical Action"=enum."Switch When Pressed", "Sub Controls"=[], "Access May Timeout"=FALSE, "Register Node"=FALSE}, {"Name"="FXP32.16", "Hidden"=FALSE, "Indicator"=FALSE, "Flattened Type"="\u0013\u0000€\u0000\u0000\u0000\u0000\u0001\u0000F@_\u0003Q\u0000 \u0000\u0000\u0000\u0010\u0000\u0001\u0000\u0001\u0000\u0000\u0000\u0010ÿÿÿÿÿÿÿÿ\u0000\u0000\u0000\u001f\u0000\u0000\u0000\u000f\u0000\u0000\u0000\u0000ÿÿÿ\u0000\u0000\u0000\u0001ÿÿÿñ\u0000\u0000\u0000\u0000\u0000\u0000\u0000\u0001\bFXP32.16\u0000\u0000\u0001\u0000\u0000\u0000\u0000\u0000\u0000\u0000\u0000\u0000\u0000\u0000\u0000\u0000\u0000", "Grouping"={"Grouped"=FALSE, "Member Names"=[], "Member IDs"=[]}, "Address"=98456, "Size"=32, "Class"=18, "Internal"=FALSE, "Typedef"={"Typedef"=FALSE, "Path"=path ""}, "ID"=38, "Bidirectional"=TRUE, "Synchronous"=FALSE, "Mechanical Action"=enum."Switch When Pressed", "Sub Controls"=[], "Access May Timeout"=FALSE, "Register Node"=FALSE}, {"Name"="FXP16.3 out", "Hidden"=FALSE, "Indicator"=TRUE, "Flattened Type"="\u0013\u0000€\u0000\u0000\u0000\u0000\u0001\u0000H@_\u0003\u0011\u0000\u0010\u0000\u0000\u0000\u0003\u0000\u0000\u0000\u0001\u0000\u0000\u0000\u0001\u0000\u0000\u0000\u0000\u0000\u0000\u0000\u0000\u0000\u0000\u0000\u0010\u0000\u0000\u0000\u0003\u0000\u0000\u0000\u0000\u0000\u0000ÿÿ\u0000\u0000\u0000\u0001ÿÿÿô\u0000\u0000\u0000\u0000\u0000\u0000\u0000\u0001\u000bFXP16.3 out\u0000\u0001\u0000\u0000\u0000\u0000\u0000\u0000\u0000\u0000\u0000\u0000\u0000\u0000\u0000\u0000", "Grouping"={"Grouped"=FALSE, "Member Names"=[], "Member IDs"=[]}, "Address"=98462, "Size"=16, "Class"=18, "Internal"=FALSE, "Typedef"={"Typedef"=FALSE, "Path"=path ""}, "ID"=39, "Bidirectional"=TRUE, "Synchronous"=FALSE, "Mechanical Action"=enum."Switch When Pressed", "Sub Controls"=[], "Access May Timeout"=FALSE, "Register Node"=FALSE}, {"Name"="FXP16.3", "Hidden"=FALSE, "Indicator"=FALSE, "Flattened Type"="\u0013\u0000€\u0000\u0000\u0000\u0000\u0001\u0000D@_\u0003\u0011\u0000\u0010\u0000\u0000\u0000\u0003\u0000\u0000\u0000\u0001\u0000\u0000\u0000\u0001\u0000\u0000\u0000\u0000\u0000\u0000\u0000\u0000\u0000\u0000\u0000\u0010\u0000\u0000\u0000\u0003\u0000\u0000\u0000\u0000\u0000\u0000ÿÿ\u0000\u0000\u0000\u0001ÿÿÿô\u0000\u0000\u0000\u0000\u0000\u0000\u0000\u0001\u0007FXP16.3\u0000\u0001\u0000\u0000\u0000\u0000\u0000\u0000\u0000\u0000\u0000\u0000\u0000\u0000\u0000\u0000", "Grouping"={"Grouped"=FALSE, "Member Names"=[], "Member IDs"=[]}, "Address"=98466, "Size"=16, "Class"=18, "Internal"=FALSE, "Typedef"={"Typedef"=FALSE, "Path"=path ""}, "ID"=40, "Bidirectional"=TRUE, "Synchronous"=FALSE, "Mechanical Action"=enum."Switch When Pressed", "Sub Controls"=[], "Access May Timeout"=FALSE, "Register Node"=FALSE}, {"Name"="FXP18.3 out", "Hidden"=FALSE, "Indicator"=TRUE, "Flattened Type"="\u0013\u0000€\u0000\u0000\u0000\u0000\u0001\u0000H@_\u0003\u0011\u0000\u0012\u0000\u0000\u0000\u0003\u0000\u0000\u0000\u0001\u0000\u0000\u0000\u0001\u0000\u0000\u0000\u0000\u0000\u0000\u0000\u0000\u0000\u0000\u0000\u0012\u0000\u0000\u0000\u0003\u0000\u0000\u0000\u0000\u0000\u0003ÿÿ\u0000\u0000\u0000\u0001ÿÿÿò\u0000\u0000\u0000\u0000\u0000\u0000\u0000\u0001\u000bFXP18.3 out\u0000\u0001\u0000\u0000\u0000\u0000\u0000\u0000\u0000\u0000\u0000\u0000\u0000\u0000\u0000\u0000", "Grouping"={"Grouped"=FALSE, "Member Names"=[], "Member IDs"=[]}, "Address"=98468, "Size"=18, "Class"=18, "Internal"=FALSE, "Typedef"={"Typedef"=FALSE, "Path"=path ""}, "ID"=41, "Bidirectional"=TRUE, "Synchronous"=FALSE, "Mechanical Action"=enum."Switch When Pressed", "Sub Controls"=[], "Access May Timeout"=FALSE, "Register Node"=FALSE}, {"Name"="FXP18.3", "Hidden"=FALSE, "Indicator"=FALSE, "Flattened Type"="\u0013\u0000€\u0000\u0000\u0000\u0000\u0001\u0000D@_\u0003\u0011\u0000\u0012\u0000\u0000\u0000\u0003\u0000\u0000\u0000\u0001\u0000\u0000\u0000\u0001\u0000\u0000\u0000\u0000\u0000\u0000\u0000\u0000\u0000\u0000\u0000\u0012\u0000\u0000\u0000\u0003\u0000\u0000\u0000\u0000\u0000\u0003ÿÿ\u0000\u0000\u0000\u0001ÿÿÿò\u0000\u0000\u0000\u0000\u0000\u0000\u0000\u0001\u0007FXP18.3\u0000\u0001\u0000\u0000\u0000\u0000\u0000\u0000\u0000\u0000\u0000\u0000\u0000\u0000\u0000\u0000", "Grouping"={"Grouped"=FALSE, "Member Names"=[], "Member IDs"=[]}, "Address"=98472, "Size"=18, "Class"=18, "Internal"=FALSE, "Typedef"={"Typedef"=FALSE, "Path"=path ""}, "ID"=42, "Bidirectional"=TRUE, "Synchronous"=FALSE, "Mechanical Action"=enum."Switch When Pressed", "Sub Controls"=[], "Access May Timeout"=FALSE, "Register Node"=FALSE}, {"Name"="Group2.FXP18.3 out", "Hidden"=FALSE, "Indicator"=TRUE, "Flattened Type"="\u0013\u0000€\u0000\u0000\u0000\u0000\u0001\u0000P@_\u0003\u0011\u0000\u0012\u0000\u0000\u0000\u0003\u0000\u0000\u0000\u0001\u0000\u0000\u0000\u0001\u0000\u0000\u0000\u0000\u0000\u0000\u0000\u0000\u0000\u0000\u0000\u0012\u0000\u0000\u0000\u0003\u0000\u0000\u0000\u0000\u0000\u0003ÿÿ\u0000\u0000\u0000\u0001ÿÿÿò\u0000\u0000\u0000\u0000\u0000\u0000\u0000\u0001\u0012Group2.FXP18.3 out\u0000\u0000\u0001\u0000\u0000\u0000\u0000\u0000\u0000\u0000\u0000\u0000\u0000\u0000\u0000\u0000\u0000", "Grouping"={"Grouped"=FALSE, "Member Names"=[], "Member IDs"=[]}, "Address"=98476, "Size"=18, "Class"=18, "Internal"=FALSE, "Typedef"={"Typedef"=FALSE, "Path"=path ""}, "ID"=43, "Bidirectional"=TRUE, "Synchronous"=FALSE, "Mechanical Action"=enum."Switch When Pressed", "Sub Controls"=[], "Access May Timeout"=FALSE, "Register Node"=FALSE}, {"Name"="Group2.FXP18.3", "Hidden"=FALSE, "Indicator"=FALSE, "Flattened Type"="\u0013\u0000€\u0000\u0000\u0000\u0000\u0001\u0000L@_\u0003\u0011\u0000\u0012\u0000\u0000\u0000\u0003\u0000\u0000\u0000\u0001\u0000\u0000\u0000\u0001\u0000\u0000\u0000\u0000\u0000\u0000\u0000\u0000\u0000\u0000\u0000\u0012\u0000\u0000\u0000\u0003\u0000\u0000\u0000\u0000\u0000\u0003ÿÿ\u0000\u0000\u0000\u0001ÿÿÿò\u0000\u0000\u0000\u0000\u0000\u0000\u0000\u0001\u000eGroup2.FXP18.3\u0000\u0000\u0001\u0000\u0000\u0000\u0000\u0000\u0000\u0000\u0000\u0000\u0000\u0000\u0000\u0000\u0000", "Grouping"={"Grouped"=FALSE, "Member Names"=[], "Member IDs"=[]}, "Address"=98480, "Size"=18, "Class"=18, "Internal"=FALSE, "Typedef"={"Typedef"=FALSE, "Path"=path ""}, "ID"=44, "Bidirectional"=TRUE, "Synchronous"=FALSE, "Mechanical Action"=enum."Switch When Pressed", "Sub Controls"=[], "Access May Timeout"=FALSE, "Register Node"=FALSE}, {"Name"="Group2.FXP16.3 out", "Hidden"=FALSE, "Indicator"=TRUE, "Flattened Type"="\u0013\u0000€\u0000\u0000\u0000\u0000\u0001\u0000P@_\u0003\u0011\u0000\u0010\u0000\u0000\u0000\u0003\u0000\u0000\u0000\u0001\u0000\u0000\u0000\u0001\u0000\u0000\u0000\u0000\u0000\u0000\u0000\u0000\u0000\u0000\u0000\u0010\u0000\u0000\u0000\u0003\u0000\u0000\u0000\u0000\u0000\u0000ÿÿ\u0000\u0000\u0000\u0001ÿÿÿô\u0000\u0000\u0000\u0000\u0000\u0000\u0000\u0001\u0012Group2.FXP16.3 out\u0000\u0000\u0001\u0000\u0000\u0000\u0000\u0000\u0000\u0000\u0000\u0000\u0000\u0000\u0000\u0000\u0000", "Grouping"={"Grouped"=FALSE, "Member Names"=[], "Member IDs"=[]}, "Address"=98486, "Size"=16, "Class"=18, "Internal"=FALSE, "Typedef"={"Typedef"=FALSE, "Path"=path ""}, "ID"=45, "Bidirectional"=TRUE, "Synchronous"=FALSE, "Mechanical Action"=enum."Switch When Pressed", "Sub Controls"=[], "Access May Timeout"=FALSE, "Register Node"=FALSE}, {"Name"="Group2.FXP16.3", "Hidden"=FALSE, "Indicator"=FALSE, "Flattened Type"="\u0013\u0000€\u0000\u0000\u0000\u0000\u0001\u0000L@_\u0003\u0011\u0000\u0010\u0000\u0000\u0000\u0003\u0000\u0000\u0000\u0001\u0000\u0000\u0000\u0001\u0000\u0000\u0000\u0000\u0000\u0000\u0000\u0000\u0000\u0000\u0000\u0010\u0000\u0000\u0000\u0003\u0000\u0000\u0000\u0000\u0000\u0000ÿÿ\u0000\u0000\u0000\u0001ÿÿÿô\u0000\u0000\u0000\u0000\u0000\u0000\u0000\u0001\u000eGroup2.FXP16.3\u0000\u0000\u0001\u0000\u0000\u0000\u0000\u0000\u0000\u0000\u0000\u0000\u0000\u0000\u0000\u0000\u0000", "Grouping"={"Grouped"=FALSE, "Member Names"=[], "Member IDs"=[]}, "Address"=98490, "Size"=16, "Class"=18, "Internal"=FALSE, "Typedef"={"Typedef"=FALSE, "Path"=path ""}, "ID"=46, "Bidirectional"=TRUE, "Synchronous"=FALSE, "Mechanical Action"=enum."Switch When Pressed", "Sub Controls"=[], "Access May Timeout"=FALSE, "Register Node"=FALSE}, {"Name"="Group2.FXP32.16 out", "Hidden"=FALSE, "Indicator"=TRUE, "Flattened Type"="\u0013\u0000€\u0000\u0000\u0000\u0000\u0001\u0000P@_\u0003Q\u0000 \u0000\u0000\u0000\u0010\u0000\u0001\u0000\u0001\u0000\u0000\u0000\u0010ÿÿÿÿÿÿÿÿ\u0000\u0000\u0000\u001f\u0000\u0000\u0000\u000f\u0000\u0000\u0000\u0000ÿÿÿ\u0000\u0000\u0000\u0001ÿÿÿñ\u0000\u0000\u0000\u0000\u0000\u0000\u0000\u0001\u0013Group2.FXP32.16 out\u0000\u0001\u0000\u0000\u0000\u0000\u0000\u0000\u0000\u0000\u0000\u0000\u0000\u0000\u0000\u0000", "Grouping"={"Grouped"=FALSE, "Member Names"=[], "Member IDs"=[]}, "Address"=98492, "Size"=32, "Class"=18, "Internal"=FALSE, "Typedef"={"Typedef"=FALSE, "Path"=path ""}, "ID"=47, "Bidirectional"=TRUE, "Synchronous"=FALSE, "Mechanical Action"=enum."Switch When Pressed", "Sub Controls"=[], "Access May Timeout"=FALSE, "Register Node"=FALSE}, {"Name"="Group2.FXP32.16", "Hidden"=FALSE, "Indicator"=FALSE, "Flattened Type"="\u0013\u0000€\u0000\u0000\u0000\u0000\u0001\u0000L@_\u0003Q\u0000 \u0000\u0000\u0000\u0010\u0000\u0001\u0000\u0001\u0000\u0000\u0000\u0010ÿÿÿÿÿÿÿÿ\u0000\u0000\u0000\u001f\u0000\u0000\u0000\u000f\u0000\u0000\u0000\u0000ÿÿÿ\u0000\u0000\u0000\u0001ÿÿÿñ\u0000\u0000\u0000\u0000\u0000\u0000\u0000\u0001\u000fGroup2.FXP32.16\u0000\u0001\u0000\u0000\u0000\u0000\u0000\u0000\u0000\u0000\u0000\u0000\u0000\u0000\u0000\u0000", "Grouping"={"Grouped"=FALSE, "Member Names"=[], "Member IDs"=[]}, "Address"=98496, "Size"=32, "Class"=18, "Internal"=FALSE, "Typedef"={"Typedef"=FALSE, "Path"=path ""}, "ID"=48, "Bidirectional"=TRUE, "Synchronous"=FALSE, "Mechanical Action"=enum."Switch When Pressed", "Sub Controls"=[], "Access May Timeout"=FALSE, "Register Node"=FALSE}, {"Name"="Group2.FXP27.5 out", "Hidden"=FALSE, "Indicator"=TRUE, "Flattened Type"="\u0013\u0000€\u0000\u0000\u0000\u0000\u0001\u0000P@_\u0003Q\u0000\u001b\u0000\u0000\u0000\u0005\u0000\u0001\u0000\u0001\u0000\u0000\u0000\u0005ÿÿÿÿÿÿÿÿ\u0000\u0000\u0000\u001a\u0000\u0000\u0000\u0004\u0000\u0000\u0000\u0000\u0003ÿÿÿ\u0000\u0000\u0000\u0001ÿÿÿë\u0000\u0000\u0000\u0000\u0000\u0000\u0000\u0001\u0012Group2.FXP27.5 out\u0000\u0000\u0001\u0000\u0000\u0000\u0000\u0000\u0000\u0000\u0000\u0000\u0000\u0000\u0000\u0000\u0000", "Grouping"={"Grouped"=FALSE, "Member Names"=[], "Member IDs"=[]}, "Address"=98500, "Size"=27, "Class"=18, "Internal"=FALSE, "Typedef"={"Typedef"=FALSE, "Path"=path ""}, "ID"=49, "Bidirectional"=TRUE, "Synchronous"=FALSE, "Mechanical Action"=enum."Switch When Pressed", "Sub Controls"=[], "Access May Timeout"=FALSE, "Register Node"=FALSE}, {"Name"="Group2.FXP27.5", "Hidden"=FALSE, "Indicator"=FALSE, "Flattened Type"="\u0013\u0000€\u0000\u0000\u0000\u0000\u0001\u0000L@_\u0003Q\u0000\u001b\u0000\u0000\u0000\u0005\u0000\u0001\u0000\u0001\u0000\u0000\u0000\u0005ÿÿÿÿÿÿÿÿ\u0000\u0000\u0000\u001a\u0000\u0000\u0000\u0004\u0000\u0000\u0000\u0000\u0003ÿÿÿ\u0000\u0000\u0000\u0001ÿÿÿë\u0000\u0000\u0000\u0000\u0000\u0000\u0000\u0001\u000eGroup2.FXP27.5\u0000\u0000\u0001\u0000\u0000\u0000\u0000\u0000\u0000\u0000\u0000\u0000\u0000\u0000\u0000\u0000\u0000", "Grouping"={"Grouped"=FALSE, "Member Names"=[], "Member IDs"=[]}, "Address"=98504, "Size"=27, "Class"=18, "Internal"=FALSE, "Typedef"={"Typedef"=FALSE, "Path"=path ""}, "ID"=50, "Bidirectional"=TRUE, "Synchronous"=FALSE, "Mechanical Action"=enum."Switch When Pressed", "Sub Controls"=[], "Access May Timeout"=FALSE, "Register Node"=FALSE}, {"Name"="Group2.FXP20.5 out", "Hidden"=FALSE, "Indicator"=TRUE, "Flattened Type"="\u0013\u0000€\u0000\u0000\u0000\u0000\u0001\u0000P@_\u0003Q\u0000\u0014\u0000\u0000\u0000\u0005\u0000\u0001\u0000\u0001\u0000\u0000\u0000\u0005ÿÿÿÿÿÿÿÿ\u0000\u0000\u0000\u0013\u0000\u0000\u0000\u0004\u0000\u0000\u0000\u0000\u0000\u0007ÿÿ\u0000\u0000\u0000\u0001ÿÿÿò\u0000\u0000\u0000\u0000\u0000\u0000\u0000\u0001\u0012Group2.FXP20.5 out\u0000\u0000\u0001\u0000\u0000\u0000\u0000\u0000\u0000\u0000\u0000\u0000\u0000\u0000\u0000\u0000\u0000", "Grouping"={"Grouped"=FALSE, "Member Names"=[], "Member IDs"=[]}, "Address"=98508, "Size"=20, "Class"=18, "Internal"=FALSE, "Typedef"={"Typedef"=FALSE, "Path"=path ""}, "ID"=51, "Bidirectional"=TRUE, "Synchronous"=FALSE, "Mechanical Action"=enum."Switch When Pressed", "Sub Controls"=[], "Access May Timeout"=FALSE, "Register Node"=FALSE}, {"Name"="Group2.FXP20.5", "Hidden"=FALSE, "Indicator"=FALSE, "Flattened Type"="\u0013\u0000€\u0000\u0000\u0000\u0000\u0001\u0000L@_\u0003Q\u0000\u0014\u0000\u0000\u0000\u0005\u0000\u0001\u0000\u0001\u0000\u0000\u0000\u0005ÿÿÿÿÿÿÿÿ\u0000\u0000\u0000\u0013\u0000\u0000\u0000\u0004\u0000\u0000\u0000\u0000\u0000\u0007ÿÿ\u0000\u0000\u0000\u0001ÿÿÿò\u0000\u0000\u0000\u0000\u0000\u0000\u0000\u0001\u000eGroup2.FXP20.5\u0000\u0000\u0001\u0000\u0000\u0000\u0000\u0000\u0000\u0000\u0000\u0000\u0000\u0000\u0000\u0000\u0000", "Grouping"={"Grouped"=FALSE, "Member Names"=[], "Member IDs"=[]}, "Address"=98512, "Size"=20, "Class"=18, "Internal"=FALSE, "Typedef"={"Typedef"=FALSE, "Path"=path ""}, "ID"=52, "Bidirectional"=TRUE, "Synchronous"=FALSE, "Mechanical Action"=enum."Switch When Pressed", "Sub Controls"=[], "Access May Timeout"=FALSE, "Register Node"=FALSE}, {"Name"="Group2.FXP16.7 out", "Hidden"=FALSE, "Indicator"=TRUE, "Flattened Type"="\u0013\u0000€\u0000\u0000\u0000\u0000\u0001\u0000P@_\u0003Q\u0000\u0010\u0000\u0000\u0000\u0007\u0000\u0001\u0000\u0001\u0000\u0000\u0000\u0007ÿÿÿÿÿÿÿÿ\u0000\u0000\u0000\u000f\u0000\u0000\u0000\u0006\u0000\u0000\u0000\u0000\u0000\u0000ÿ\u0000\u0000\u0000\u0001ÿÿÿø\u0000\u0000\u0000\u0000\u0000\u0000\u0000\u0001\u0012Group2.FXP16.7 out\u0000\u0000\u0001\u0000\u0000\u0000\u0000\u0000\u0000\u0000\u0000\u0000\u0000\u0000\u0000\u0000\u0000", "Grouping"={"Grouped"=FALSE, "Member Names"=[], "Member IDs"=[]}, "Address"=98518, "Size"=16, "Class"=18, "Internal"=FALSE, "Typedef"={"Typedef"=FALSE, "Path"=path ""}, "ID"=53, "Bidirectional"=TRUE, "Synchronous"=FALSE, "Mechanical Action"=enum."Switch When Pressed", "Sub Controls"=[], "Access May Timeout"=FALSE, "Register Node"=FALSE}, {"Name"="Group2.FXP16.7", "Hidden"=FALSE, "Indicator"=FALSE, "Flattened Type"="\u0013\u0000€\u0000\u0000\u0000\u0000\u0001\u0000L@_\u0003Q\u0000\u0010\u0000\u0000\u0000\u0007\u0000\u0001\u0000\u0001\u0000\u0000\u0000\u0007ÿÿÿÿÿÿÿÿ\u0000\u0000\u0000\u000f\u0000\u0000\u0000\u0006\u0000\u0000\u0000\u0000\u0000\u0000ÿ\u0000\u0000\u0000\u0001ÿÿÿø\u0000\u0000\u0000\u0000\u0000\u0000\u0000\u0001\u000eGroup2.FXP16.7\u0000\u0000\u0001\u0000\u0000\u0000\u0000\u0000\u0000\u0000\u0000\u0000\u0000\u0000\u0000\u0000\u0000", "Grouping"={"Grouped"=FALSE, "Member Names"=[], "Member IDs"=[]}, "Address"=98522, "Size"=16, "Class"=18, "Internal"=FALSE, "Typedef"={"Typedef"=FALSE, "Path"=path ""}, "ID"=54, "Bidirectional"=TRUE, "Synchronous"=FALSE, "Mechanical Action"=enum."Switch When Pressed", "Sub Controls"=[], "Access May Timeout"=FALSE, "Register Node"=FALSE}, {"Name"="Group2.FXP64.32 out", "Hidden"=FALSE, "Indicator"=TRUE, "Flattened Type"="\u0013\u0000€\u0000\u0000\u0000\u0000\u0001\u0000P@_\u0003Q\u0000@\u0000\u0000\u0000 \u0000\u0001\u0000\u0001\u0000\u0000\u0000 ÿÿÿÿÿÿÿÿ\u0000\u0000\u0000?\u0000\u0000\u0000\u001fÿÿÿÿÿÿÿ\u0000\u0000\u0000\u0001ÿÿÿá\u0000\u0000\u0000\u0000\u0000\u0000\u0000\u0001\u0013Group2.FXP64.32 out\u0000\u0001\u0000\u0000\u0000\u0000\u0000\u0000\u0000\u0000\u0000\u0000\u0000\u0000\u0000\u0000", "Grouping"={"Grouped"=FALSE, "Member Names"=[], "Member IDs"=[]}, "Address"=98524, "Size"=64, "Class"=18, "Internal"=FALSE, "Typedef"={"Typedef"=FALSE, "Path"=path ""}, "ID"=55, "Bidirectional"=TRUE, "Synchronous"=FALSE, "Mechanical Action"=enum."Switch When Pressed", "Sub Controls"=[], "Access May Timeout"=FALSE, "Register Node"=FALSE}, {"Name"="Group2.FXP32.8 out", "Hidden"=FALSE, "Indicator"=TRUE, "Flattened Type"="\u0013\u0000€\u0000\u0000\u0000\u0000\u0001\u0000P@_\u0003Q\u0000 \u0000\u0000\u0000\b\u0000\u0001\u0000\u0001\u0000\u0000\u0000\bÿÿÿÿÿÿÿÿ\u0000\u0000\u0000\u001f\u0000\u0000\u0000\u0007\u0000\u0000\u0000\u0000ÿÿÿ\u0000\u0000\u0000\u0001ÿÿÿé\u0000\u0000\u0000\u0000\u0000\u0000\u0000\u0001\u0012Group2.FXP32.8 out\u0000\u0000\u0001\u0000\u0000\u0000\u0000\u0000\u0000\u0000\u0000\u0000\u0000\u0000\u0000\u0000\u0000", "Grouping"={"Grouped"=FALSE, "Member Names"=[], "Member IDs"=[]}, "Address"=98528, "Size"=32, "Class"=18, "Internal"=FALSE, "Typedef"={"Typedef"=FALSE, "Path"=path ""}, "ID"=56, "Bidirectional"=TRUE, "Synchronous"=FALSE, "Mechanical Action"=enum."Switch When Pressed", "Sub Controls"=[], "Access May Timeout"=FALSE, "Register Node"=FALSE}, {"Name"="Group2.FXP16.5 out", "Hidden"=FALSE, "Indicator"=TRUE, "Flattened Type"="\u0013\u0000€\u0000\u0000\u0000\u0000\u0001\u0000P@_\u0003Q\u0000\u0010\u0000\u0000\u0000\u0005\u0000\u0001\u0000\u0001\u0000\u0000\u0000\u0005ÿÿÿÿÿÿÿÿ\u0000\u0000\u0000\u000f\u0000\u0000\u0000\u0004\u0000\u0000\u0000\u0000\u0000\u0000ÿ\u0000\u0000\u0000\u0001ÿÿÿö\u0000\u0000\u0000\u0000\u0000\u0000\u0000\u0001\u0012Group2.FXP16.5 out\u0000\u0000\u0001\u0000\u0000\u0000\u0000\u0000\u0000\u0000\u0000\u0000\u0000\u0000\u0000\u0000\u0000", "Grouping"={"Grouped"=FALSE, "Member Names"=[], "Member IDs"=[]}, "Address"=98534, "Size"=16, "Class"=18, "Internal"=FALSE, "Typedef"={"Typedef"=FALSE, "Path"=path ""}, "ID"=57, "Bidirectional"=TRUE, "Synchronous"=FALSE, "Mechanical Action"=enum."Switch When Pressed", "Sub Controls"=[], "Access May Timeout"=FALSE, "Register Node"=FALSE}, {"Name"="Group2.FXP24.5 out", "Hidden"=FALSE, "Indicator"=TRUE, "Flattened Type"="\u0013\u0000€\u0000\u0000\u0000\u0000\u0001\u0000P@_\u0003Q\u0000\u0018\u0000\u0000\u0000\u0005\u0000\u0001\u0000\u0001\u0000\u0000\u0000\u0005ÿÿÿÿÿÿÿÿ\u0000\u0000\u0000\u0017\u0000\u0000\u0000\u0004\u0000\u0000\u0000\u0000\u0000ÿÿ\u0000\u0000\u0000\u0001ÿÿÿî\u0000\u0000\u0000\u0000\u0000\u0000\u0000\u0001\u0012Group2.FXP24.5 out\u0000\u0000\u0001\u0000\u0000\u0000\u0000\u0000\u0000\u0000\u0000\u0000\u0000\u0000\u0000\u0000\u0000", "Grouping"={"Grouped"=FALSE, "Member Names"=[], "Member IDs"=[]}, "Address"=98536, "Size"=24, "Class"=18, "Internal"=FALSE, "Typedef"={"Typedef"=FALSE, "Path"=path ""}, "ID"=58, "Bidirectional"=TRUE, "Synchronous"=FALSE, "Mechanical Action"=enum."Switch When Pressed", "Sub Controls"=[], "Access May Timeout"=FALSE, "Register Node"=FALSE}, {"Name"="Group2.FXP64.32", "Hidden"=FALSE, "Indicator"=FALSE, "Flattened Type"="\u0013\u0000€\u0000\u0000\u0000\u0000\u0001\u0000L@_\u0003Q\u0000@\u0000\u0000\u0000 \u0000\u0001\u0000\u0001\u0000\u0000\u0000 ÿÿÿÿÿÿÿÿ\u0000\u0000\u0000?\u0000\u0000\u0000\u001fÿÿÿÿÿÿÿ\u0000\u0000\u0000\u0001ÿÿÿá\u0000\u0000\u0000\u0000\u0000\u0000\u0000\u0001\u000fGroup2.FXP64.32\u0000\u0001\u0000\u0000\u0000\u0000\u0000\u0000\u0000\u0000\u0000\u0000\u0000\u0000\u0000\u0000", "Grouping"={"Grouped"=FALSE, "Member Names"=[], "Member IDs"=[]}, "Address"=98540, "Size"=64, "Class"=18, "Internal"=FALSE, "Typedef"={"Typedef"=FALSE, "Path"=path ""}, "ID"=59, "Bidirectional"=TRUE, "Synchronous"=FALSE, "Mechanical Action"=enum."Switch When Pressed", "Sub Controls"=[], "Access May Timeout"=FALSE, "Register Node"=FALSE}, {"Name"="Group2.FXP32.8", "Hidden"=FALSE, "Indicator"=FALSE, "Flattened Type"="\u0013\u0000€\u0000\u0000\u0000\u0000\u0001\u0000L@_\u0003Q\u0000 \u0000\u0000\u0000\b\u0000\u0001\u0000\u0001\u0000\u0000\u0000\bÿÿÿÿÿÿÿÿ\u0000\u0000\u0000\u001f\u0000\u0000\u0000\u0007\u0000\u0000\u0000\u0000ÿÿÿ\u0000\u0000\u0000\u0001ÿÿÿé\u0000\u0000\u0000\u0000\u0000\u0000\u0000\u0001\u000eGroup2.FXP32.8\u0000\u0000\u0001\u0000\u0000\u0000\u0000\u0000\u0000\u0000\u0000\u0000\u0000\u0000\u0000\u0000\u0000", "Grouping"={"Grouped"=FALSE, "Member Names"=[], "Member IDs"=[]}, "Address"=98544, "Size"=32, "Class"=18, "Internal"=FALSE, "Typedef"={"Typedef"=FALSE, "Path"=path ""}, "ID"=60, "Bidirectional"=TRUE, "Synchronous"=FALSE, "Mechanical Action"=enum."Switch When Pressed", "Sub Controls"=[], "Access May Timeout"=FALSE, "Register Node"=FALSE}, {"Name"="Group2.FXP16.5", "Hidden"=FALSE, "Indicator"=FALSE, "Flattened Type"="\u0013\u0000€\u0000\u0000\u0000\u0000\u0001\u0000L@_\u0003Q\u0000\u0010\u0000\u0000\u0000\u0005\u0000\u0001\u0000\u0001\u0000\u0000\u0000\u0005ÿÿÿÿÿÿÿÿ\u0000\u0000\u0000\u000f\u0000\u0000\u0000\u0004\u0000\u0000\u0000\u0000\u0000\u0000ÿ\u0000\u0000\u0000\u0001ÿÿÿö\u0000\u0000\u0000\u0000\u0000\u0000\u0000\u0001\u000eGroup2.FXP16.5\u0000\u0000\u0001\u0000\u0000\u0000\u0000\u0000\u0000\u0000\u0000\u0000\u0000\u0000\u0000\u0000\u0000", "Grouping"={"Grouped"=FALSE, "Member Names"=[], "Member IDs"=[]}, "Address"=98550, "Size"=16, "Class"=18, "Internal"=FALSE, "Typedef"={"Typedef"=FALSE, "Path"=path ""}, "ID"=61, "Bidirectional"=TRUE, "Synchronous"=FALSE, "Mechanical Action"=enum."Switch When Pressed", "Sub Controls"=[], "Access May Timeout"=FALSE, "Register Node"=FALSE}, {"Name"="Group2.FXP24.5", "Hidden"=FALSE, "Indicator"=FALSE, "Flattened Type"="\u0013\u0000€\u0000\u0000\u0000\u0000\u0001\u0000L@_\u0003Q\u0000\u0018\u0000\u0000\u0000\u0005\u0000\u0001\u0000\u0001\u0000\u0000\u0000\u0005ÿÿÿÿÿÿÿÿ\u0000\u0000\u0000\u0017\u0000\u0000\u0000\u0004\u0000\u0000\u0000\u0000\u0000ÿÿ\u0000\u0000\u0000\u0001ÿÿÿî\u0000\u0000\u0000\u0000\u0000\u0000\u0000\u0001\u000eGroup2.FXP24.5\u0000\u0000\u0001\u0000\u0000\u0000\u0000\u0000\u0000\u0000\u0000\u0000\u0000\u0000\u0000\u0000\u0000", "Grouping"={"Grouped"=FALSE, "Member Names"=[], "Member IDs"=[]}, "Address"=98552, "Size"=24, "Class"=18, "Internal"=FALSE, "Typedef"={"Typedef"=FALSE, "Path"=path ""}, "ID"=62, "Bidirectional"=TRUE, "Synchronous"=FALSE, "Mechanical Action"=enum."Switch When Pressed", "Sub Controls"=[], "Access May Timeout"=FALSE, "Register Node"=FALSE}, {"Name"="Group2.Boolean out", "Hidden"=FALSE, "Indicator"=TRUE, "Flattened Type"="\u0013\u0000€\u0000\u0000\u0000\u0000\u0001\u0000\u0018@!\u0012Group2.Boolean out\u0000\u0000\u0001\u0000\u0000\u0000\u0000\u0000\u0000\u0000", "Grouping"={"Grouped"=FALSE, "Member Names"=[], "Member IDs"=[]}, "Address"=98558, "Size"=1, "Class"=8, "Internal"=FALSE, "Typedef"={"Typedef"=FALSE, "Path"=path ""}, "ID"=63, "Bidirectional"=TRUE, "Synchronous"=FALSE, "Mechanical Action"=enum."Switch When Pressed", "Sub Controls"=[], "Access May Timeout"=FALSE, "Register Node"=FALSE}, {"Name"="Group1.SGL out", "Hidden"=FALSE, "Indicator"=TRUE, "Flattened Type"="\u0013\u0000€\u0000\u0000\u0000\u0000\u0001\u0000\u0015@\t\u0000\u000eGroup1.SGL out\u0000\u0000\u0001\u0000\u0000\u0000\u0000\u0000\u0000\u0000\u0000\u0000\u0000", "Grouping"={"Grouped"=FALSE, "Member Names"=[], "Member IDs"=[]}, "Address"=98560, "Size"=32, "Class"=18, "Internal"=FALSE, "Typedef"={"Typedef"=FALSE, "Path"=path ""}, "ID"=64, "Bidirectional"=TRUE, "Synchronous"=FALSE, "Mechanical Action"=enum."Switch When Pressed", "Sub Controls"=[], "Access May Timeout"=FALSE, "Register Node"=FALSE}, {"Name"="Group1.U32 out", "Hidden"=FALSE, "Indicator"=TRUE, "Flattened Type"="\u0013\u0000€\u0000\u0000\u0000\u0000\u0001\u0000\u0015@\u0007\u0000\u000eGroup1.U32 out\u0000\u0000\u0001\u0000\u0000\u0000\u0000\u0000\u0000\u0000\u0000\u0000\u0000", "Grouping"={"Grouped"=FALSE, "Member Names"=[], "Member IDs"=[]}, "Address"=98564, "Size"=32, "Class"=18, "Internal"=FALSE, "Typedef"={"Typedef"=FALSE, "Path"=path ""}, "ID"=65, "Bidirectional"=TRUE, "Synchronous"=FALSE, "Mechanical Action"=enum."Switch When Pressed", "Sub Controls"=[], "Access May Timeout"=FALSE, "Register Node"=FALSE}, {"Name"="Group1.U64 out", "Hidden"=FALSE, "Indicator"=TRUE, "Flattened Type"="\u0013\u0000€\u0000\u0000\u0000\u0000\u0001\u0000\u0015@\b\u0000\u000eGroup1.U64 out\u0000\u0000\u0001\u0000\u0000\u0000\u0000\u0000\u0000\u0000\u0000\u0000\u0000\u0000\u0000\u0000\u0000", "Grouping"={"Grouped"=FALSE, "Member Names"=[], "Member IDs"=[]}, "Address"=98568, "Size"=64, "Class"=18, "Internal"=FALSE, "Typedef"={"Typedef"=FALSE, "Path"=path ""}, "ID"=66, "Bidirectional"=TRUE, "Synchronous"=FALSE, "Mechanical Action"=enum."Switch When Pressed", "Sub Controls"=[], "Access May Timeout"=FALSE, "Register Node"=FALSE}, {"Name"="Group1.U8 out", "Hidden"=FALSE, "Indicator"=TRUE, "Flattened Type"="\u0013\u0000€\u0000\u0000\u0000\u0000\u0001\u0000\u0013@\u0005\u0000\rGroup1.U8 out\u0000\u0001\u0000\u0000\u0000\u0000\u0000\u0000\u0000", "Grouping"={"Grouped"=FALSE, "Member Names"=[], "Member IDs"=[]}, "Address"=98574, "Size"=8, "Class"=18, "Internal"=FALSE, "Typedef"={"Typedef"=FALSE, "Path"=path ""}, "ID"=67, "Bidirectional"=TRUE, "Synchronous"=FALSE, "Mechanical Action"=enum."Switch When Pressed", "Sub Controls"=[], "Access May Timeout"=FALSE, "Register Node"=FALSE}, {"Name"="Group1.U16 out", "Hidden"=FALSE, "Indicator"=TRUE, "Flattened Type"="\u0013\u0000€\u0000\u0000\u0000\u0000\u0001\u0000\u0015@\u0006\u0000\u000eGroup1.U16 out\u0000\u0000\u0001\u0000\u0000\u0000\u0000\u0000\u0000\u0000\u0000", "Grouping"={"Grouped"=FALSE, "Member Names"=[], "Member IDs"=[]}, "Address"=98578, "Size"=16, "Class"=18, "Internal"=FALSE, "Typedef"={"Typedef"=FALSE, "Path"=path ""}, "ID"=68, "Bidirectional"=TRUE, "Synchronous"=FALSE, "Mechanical Action"=enum."Switch When Pressed", "Sub Controls"=[], "Access May Timeout"=FALSE, "Register Node"=FALSE}, {"Name"="Group1.I32 out", "Hidden"=FALSE, "Indicator"=TRUE, "Flattened Type"="\u0013\u0000€\u0000\u0000\u0000\u0000\u0001\u0000\u0015@\u0003\u0000\u000eGroup1.I32 out\u0000\u0000\u0001\u0000\u0000\u0000\u0000\u0000\u0000\u0000\u0000\u0000\u0000", "Grouping"={"Grouped"=FALSE, "Member Names"=[], "Member IDs"=[]}, "Address"=98580, "Size"=32, "Class"=18, "Internal"=FALSE, "Typedef"={"Typedef"=FALSE, "Path"=path ""}, "ID"=69, "Bidirectional"=TRUE, "Synchronous"=FALSE, "Mechanical Action"=enum."Switch When Pressed", "Sub Controls"=[], "Access May Timeout"=FALSE, "Register Node"=FALSE}, {"Name"="Group1.I64 out", "Hidden"=FALSE, "Indicator"=TRUE, "Flattened Type"="\u0013\u0000€\u0000\u0000\u0000\u0000\u0001\u0000\u0015@\u0004\u0000\u000eGroup1.I64 out\u0000\u0000\u0001\u0000\u0000\u0000\u0000\u0000\u0000\u0000\u0000\u0000\u0000\u0000\u0000\u0000\u0000", "Grouping"={"Grouped"=FALSE, "Member Names"=[], "Member IDs"=[]}, "Address"=98584, "Size"=64, "Class"=18, "Internal"=FALSE, "Typedef"={"Typedef"=FALSE, "Path"=path ""}, "ID"=70, "Bidirectional"=TRUE, "Synchronous"=FALSE, "Mechanical Action"=enum."Switch When Pressed", "Sub Controls"=[], "Access May Timeout"=FALSE, "Register Node"=FALSE}, {"Name"="Group1.I8 out", "Hidden"=FALSE, "Indicator"=TRUE, "Flattened Type"="\u0013\u0000€\u0000\u0000\u0000\u0000\u0001\u0000\u0013@\u0001\u0000\rGroup1.I8 out\u0000\u0001\u0000\u0000\u0000\u0000\u0000\u0000\u0000", "Grouping"={"Grouped"=FALSE, "Member Names"=[], "Member IDs"=[]}, "Address"=98590, "Size"=8, "Class"=18, "Internal"=FALSE, "Typedef"={"Typedef"=FALSE, "Path"=path ""}, "ID"=71, "Bidirectional"=TRUE, "Synchronous"=FALSE, "Mechanical Action"=enum."Switch When Pressed", "Sub Controls"=[], "Access May Timeout"=FALSE, "Register Node"=FALSE}, {"Name"="Group1.I16 out", "Hidden"=FALSE, "Indicator"=TRUE, "Flattened Type"="\u0013\u0000€\u0000\u0000\u0000\u0000\u0001\u0000\u0015@\u0002\u0000\u000eGroup1.I16 out\u0000\u0000\u0001\u0000\u0000\u0000\u0000\u0000\u0000\u0000\u0000", "Grouping"={"Grouped"=FALSE, "Member Names"=[], "Member IDs"=[]}, "Address"=98594, "Size"=16, "Class"=18, "Internal"=FALSE, "Typedef"={"Typedef"=FALSE, "Path"=path ""}, "ID"=72, "Bidirectional"=TRUE, "Synchronous"=FALSE, "Mechanical Action"=enum."Switch When Pressed", "Sub Controls"=[], "Access May Timeout"=FALSE, "Register Node"=FALSE}, {"Name"="Group2.Boolean", "Hidden"=FALSE, "Indicator"=FALSE, "Flattened Type"="\u0013\u0000€\u0000\u0000\u0000\u0000\u0001\u0000\u0014@!\u000eGroup2.Boolean\u0000\u0000\u0001\u0000\u0000\u0000\u0000\u0000\u0000\u0000", "Grouping"={"Grouped"=FALSE, "Member Names"=[], "Member IDs"=[]}, "Address"=98598, "Size"=1, "Class"=8, "Internal"=FALSE, "Typedef"={"Typedef"=FALSE, "Path"=path ""}, "ID"=73, "Bidirectional"=TRUE, "Synchronous"=FALSE, "Mechanical Action"=enum."Switch When Pressed", "Sub Controls"=[], "Access May Timeout"=FALSE, "Register Node"=FALSE}, {"Name"="Group1.SGL", "Hidden"=FALSE, "Indicator"=FALSE, "Flattened Type"="\u0013\u0000€\u0000\u0000\u0000\u0000\u0001\u0000\u0011@\t\u0000\nGroup1.SGL\u0000\u0000\u0001\u0000\u0000\u0000\u0000\u0000\u0000\u0000\u0000\u0000\u0000", "Grouping"={"Grouped"=FALSE, "Member Names"=[], "Member IDs"=[]}, "Address"=98600, "Size"=32, "Class"=18, "Internal"=FALSE, "Typedef"={"Typedef"=FALSE, "Path"=path ""}, "ID"=74, "Bidirectional"=TRUE, "Synchronous"=FALSE, "Mechanical Action"=enum."Switch When Pressed", "Sub Controls"=[], "Access May Timeout"=FALSE, "Register Node"=FALSE}, {"Name"="Group1.U32", "Hidden"=FALSE, "Indicator"=FALSE, "Flattened Type"="\u0013\u0000€\u0000\u0000\u0000\u0000\u0001\u0000\u0011@\u0007\u0000\nGroup1.U32\u0000\u0000\u0001\u0000\u0000\u0000\u0000\u0000\u0000\u0000\u0000\u0000\u0000", "Grouping"={"Grouped"=FALSE, "Member Names"=[], "Member IDs"=[]}, "Address"=98604, "Size"=32, "Class"=18, "Internal"=FALSE, "Typedef"={"Typedef"=FALSE, "Path"=path ""}, "ID"=75, "Bidirectional"=TRUE, "Synchronous"=FALSE, "Mechanical Action"=enum."Switch When Pressed", "Sub Controls"=[], "Access May Timeout"=FALSE, "Register Node"=FALSE}, {"Name"="Group1.U64", "Hidden"=FALSE, "Indicator"=FALSE, "Flattened Type"="\u0013\u0000€\u0000\u0000\u0000\u0000\u0001\u0000\u0011@\b\u0000\nGroup1.U64\u0000\u0000\u0001\u0000\u0000\u0000\u0000\u0000\u0000\u0000\u0000\u0000\u0000\u0000\u0000\u0000\u0000", "Grouping"={"Grouped"=FALSE, "Member Names"=[], "Member IDs"=[]}, "Address"=98608, "Size"=64, "Class"=18, "Internal"=FALSE, "Typedef"={"Typedef"=FALSE, "Path"=path ""}, "ID"=76, "Bidirectional"=TRUE, "Synchronous"=FALSE, "Mechanical Action"=enum."Switch When Pressed", "Sub Controls"=[], "Access May Timeout"=FALSE, "Register Node"=FALSE}, {"Name"="Group1.U8", "Hidden"=FALSE, "Indicator"=FALSE, "Flattened Type"="\u0013\u0000€\u0000\u0000\u0000\u0000\u0001\u0000\u000f@\u0005\u0000\tGroup1.U8\u0000\u0001\u0000\u0000\u0000\u0000\u0000\u0000\u0000", "Grouping"={"Grouped"=FALSE, "Member Names"=[], "Member IDs"=[]}, "Address"=98614, "Size"=8, "Class"=18, "Internal"=FALSE, "Typedef"={"Typedef"=FALSE, "Path"=path ""}, "ID"=77, "Bidirectional"=TRUE, "Synchronous"=FALSE, "Mechanical Action"=enum."Switch When Pressed", "Sub Controls"=[], "Access May Timeout"=FALSE, "Register Node"=FALSE}, {"Name"="Group1.U16", "Hidden"=FALSE, "Indicator"=FALSE, "Flattened Type"="\u0013\u0000€\u0000\u0000\u0000\u0000\u0001\u0000\u0011@\u0006\u0000\nGroup1.U16\u0000\u0000\u0001\u0000\u0000\u0000\u0000\u0000\u0000\u0000\u0000", "Grouping"={"Grouped"=FALSE, "Member Names"=[], "Member IDs"=[]}, "Address"=98618, "Size"=16, "Class"=18, "Internal"=FALSE, "Typedef"={"Typedef"=FALSE, "Path"=path ""}, "ID"=78, "Bidirectional"=TRUE, "Synchronous"=FALSE, "Mechanical Action"=enum."Switch When Pressed", "Sub Controls"=[], "Access May Timeout"=FALSE, "Register Node"=FALSE}, {"Name"="Group1.I32", "Hidden"=FALSE, "Indicator"=FALSE, "Flattened Type"="\u0013\u0000€\u0000\u0000\u0000\u0000\u0001\u0000\u0011@\u0003\u0000\nGroup1.I32\u0000\u0000\u0001\u0000\u0000\u0000\u0000\u0000\u0000\u0000\u0000\u0000\u0000", "Grouping"={"Grouped"=FALSE, "Member Names"=[], "Member IDs"=[]}, "Address"=98620, "Size"=32, "Class"=18, "Internal"=FALSE, "Typedef"={"Typedef"=FALSE, "Path"=path ""}, "ID"=79, "Bidirectional"=TRUE, "Synchronous"=FALSE, "Mechanical Action"=enum."Switch When Pressed", "Sub Controls"=[], "Access May Timeout"=FALSE, "Register Node"=FALSE}, {"Name"="Group1.I64", "Hidden"=FALSE, "Indicator"=FALSE, "Flattened Type"="\u0013\u0000€\u0000\u0000\u0000\u0000\u0001\u0000\u0011@\u0004\u0000\nGroup1.I64\u0000\u0000\u0001\u0000\u0000\u0000\u0000\u0000\u0000\u0000\u0000\u0000\u0000\u0000\u0000\u0000\u0000", "Grouping"={"Grouped"=FALSE, "Member Names"=[], "Member IDs"=[]}, "Address"=98624, "Size"=64, "Class"=18, "Internal"=FALSE, "Typedef"={"Typedef"=FALSE, "Path"=path ""}, "ID"=80, "Bidirectional"=TRUE, "Synchronous"=FALSE, "Mechanical Action"=enum."Switch When Pressed", "Sub Controls"=[], "Access May Timeout"=FALSE, "Register Node"=FALSE}, {"Name"="Group1.I8", "Hidden"=FALSE, "Indicator"=FALSE, "Flattened Type"="\u0013\u0000€\u0000\u0000\u0000\u0000\u0001\u0000\u000f@\u0001\u0000\tGroup1.I8\u0000\u0001\u0000\u0000\u0000\u0000\u0000\u0000\u0000", "Grouping"={"Grouped"=FALSE, "Member Names"=[], "Member IDs"=[]}, "Address"=98630, "Size"=8, "Class"=18, "Internal"=FALSE, "Typedef"={"Typedef"=FALSE, "Path"=path ""}, "ID"=81, "Bidirectional"=TRUE, "Synchronous"=FALSE, "Mechanical Action"=enum."Switch When Pressed", "Sub Controls"=[], "Access May Timeout"=FALSE, "Register Node"=FALSE}, {"Name"="Group1.I16", "Hidden"=FALSE, "Indicator"=FALSE, "Flattened Type"="\u0013\u0000€\u0000\u0000\u0000\u0000\u0001\u0000\u0011@\u0002\u0000\nGroup1.I16\u0000\u0000\u0001\u0000\u0000\u0000\u0000\u0000\u0000\u0000\u0000", "Grouping"={"Grouped"=FALSE, "Member Names"=[], "Member IDs"=[]}, "Address"=98634, "Size"=16, "Class"=18, "Internal"=FALSE, "Typedef"={"Typedef"=FALSE, "Path"=path ""}, "ID"=82, "Bidirectional"=TRUE, "Synchronous"=FALSE, "Mechanical Action"=enum."Switch When Pressed", "Sub Controls"=[], "Access May Timeout"=FALSE, "Register Node"=FALSE}, {"Name"="Fast timeout 2", "Hidden"=FALSE, "Indicator"=TRUE, "Flattened Type"="\u0013\u0000€\u0000\u0000\u0000\u0000\u0001\u0000\u0014@!\u000eFast timeout 2\u0000\u0000\u0001\u0000\u0000\u0000\u0000\u0000\u0000\u0000", "Grouping"={"Grouped"=FALSE, "Member Names"=[], "Member IDs"=[]}, "Address"=98638, "Size"=1, "Class"=8, "Internal"=FALSE, "Typedef"={"Typedef"=FALSE, "Path"=path ""}, "ID"=83, "Bidirectional"=TRUE, "Synchronous"=FALSE, "Mechanical Action"=enum."Switch When Pressed", "Sub Controls"=[], "Access May Timeout"=FALSE, "Register Node"=FALSE}, {"Name"="Fast timeout 3", "Hidden"=FALSE, "Indicator"=TRUE, "Flattened Type"="\u0013\u0000€\u0000\u0000\u0000\u0000\u0001\u0000\u0014@!\u000eFast timeout 3\u0000\u0000\u0001\u0000\u0000\u0000\u0000\u0000\u0000\u0000", "Grouping"={"Grouped"=FALSE, "Member Names"=[], "Member IDs"=[]}, "Address"=98642, "Size"=1, "Class"=8, "Internal"=FALSE, "Typedef"={"Typedef"=FALSE, "Path"=path ""}, "ID"=84, "Bidirectional"=TRUE, "Synchronous"=FALSE, "Mechanical Action"=enum."Switch When Pressed", "Sub Controls"=[], "Access May Timeout"=FALSE, "Register Node"=FALSE}, {"Name"="ViControl", "Hidden"=FALSE, "Indicator"=FALSE, "Flattened Type"="", "Grouping"={"Grouped"=FALSE, "Member Names"=[], "Member IDs"=[]}, "Address"=94208, "Size"=32, "Class"=0, "Internal"=TRUE, "Typedef"={"Typedef"=FALSE, "Path"=path ""}, "ID"=0, "Bidirectional"=TRUE, "Synchronous"=FALSE, "Mechanical Action"=enum."Switch When Pressed", "Sub Controls"=[], "Access May Timeout"=FALSE, "Register Node"=FALSE}, {"Name"="DiagramReset", "Hidden"=FALSE, "Indicator"=FALSE, "Flattened Type"="", "Grouping"={"Grouped"=FALSE, "Member Names"=[], "Member IDs"=[]}, "Address"=94216, "Size"=32, "Class"=0, "Internal"=TRUE, "Typedef"={"Typedef"=FALSE, "Path"=path ""}, "ID"=0, "Bidirectional"=TRUE, "Synchronous"=FALSE, "Mechanical Action"=enum."Switch When Pressed", "Sub Controls"=[], "Access May Timeout"=FALSE, "Register Node"=FALSE}, {"Name"="ViSignature", "Hidden"=TRUE, "Indicator"=TRUE, "Flattened Type"="", "Grouping"={"Grouped"=FALSE, "Member Names"=[], "Member IDs"=[]}, "Address"=94212, "Size"=128, "Class"=0, "Internal"=TRUE, "Typedef"={"Typedef"=FALSE, "Path"=path ""}, "ID"=0, "Bidirectional"=FALSE, "Synchronous"=FALSE, "Mechanical Action"=enum."Switch When Pressed", "Sub Controls"=[], "Access May Timeout"=FALSE, "Register Node"=FALSE}, {"Name"="InterruptEnable", "Hidden"=FALSE, "Indicator"=FALSE, "Flattened Type"="", "Grouping"={"Grouped"=FALSE, "Member Names"=[], "Member IDs"=[]}, "Address"=90112, "Size"=32, "Class"=0, "Internal"=TRUE, "Typedef"={"Typedef"=FALSE, "Path"=path ""}, "ID"=0, "Bidirectional"=TRUE, "Synchronous"=FALSE, "Mechanical Action"=enum."Switch When Pressed", "Sub Controls"=[], "Access May Timeout"=FALSE, "Register Node"=FALSE}, {"Name"="InterruptMask", "Hidden"=FALSE, "Indicator"=FALSE, "Flattened Type"="", "Grouping"={"Grouped"=FALSE, "Member Names"=[], "Member IDs"=[]}, "Address"=90120, "Size"=32, "Class"=0, "Internal"=TRUE, "Typedef"={"Typedef"=FALSE, "Path"=path ""}, "ID"=0, "Bidirectional"=TRUE, "Synchronous"=FALSE, "Mechanical Action"=enum."Switch When Pressed", "Sub Controls"=[], "Access May Timeout"=FALSE, "Register Node"=FALSE}, {"Name"="InterruptStatus", "Hidden"=FALSE, "Indicator"=FALSE, "Flattened Type"="", "Grouping"={"Grouped"=FALSE, "Member Names"=[], "Member IDs"=[]}, "Address"=90124, "Size"=32, "Class"=0, "Internal"=TRUE, "Typedef"={"Typedef"=FALSE, "Path"=path ""}, "ID"=0, "Bidirectional"=TRUE, "Synchronous"=FALSE, "Mechanical Action"=enum."Switch When Pressed", "Sub Controls"=[], "Access May Timeout"=FALSE, "Register Node"=FALSE}]  # Expected Available Registers
      # "Assert the correct array of available DMAs"
      # "Assert the correct array of available registers"
      n2 = call "Generate cRIO-9068 Bitfile Path.vi"() -> ("Bitfile Path"=w5:path)
      n3 = call "Parse FPGA Bitfile.vi"("error in (no error)"=w16, "Path"=w5) -> ("error out"=w15:errorcluster, "DMA configuration array"=w9:T1[], "vi info"=w14:T9)  [unwired: 7 in]
      n4 = Unbundle By Name(w14) -> ("RegisterMap"=w13:T4[])
      n5 = call-dynamic "passIfEqual.vi"("error in (no error)"=w15, "y"=w13, "x"=w6, "TestCase in"=w17) -> ("error out"=w11:errorcluster, "TestCase out"=w8:refnum<class "Load And Parse Bitfile Testing.lvclass">)  [unwired: 6 in]
      n6 = call-dynamic "passIfEqual.vi"("error in (no error)"=w11, "y"=w9, "x"=w7, "TestCase in"=w8) -> ("error out"=w10:errorcluster, "TestCase out"=w12:refnum<class "Load And Parse Bitfile Testing.lvclass">)  [unwired: 6 in]
    }
    frame Disabled {
      # "skip test result while test is under development"
      n7 = call <vilib>:"skip.vi"("error in (no error)"=w18, "TestCase in"=w21) -> ("error out"=w20:errorcluster, "TestCase out"=w19:refnum<class "Load And Parse Bitfile Testing.lvclass">)  [unwired: 8 in]
    }
  }
  "error out" <- w3
  "TestCase out" <- w1
